vi "op_ClearNoise.vi"(0 "EQ folder path Refnum":refnum<vi>, 1 "HV enable button":bool caption="High Voltage enable", 2 "HV parameters Refnum":refnum<vi>, 3 "HV level Refnum":refnum<vi>, 4 "HV string Refnum":refnum<vi>, 5 "Stop ACQ button Refnum":refnum<vi>, 6 "ACQ Parameters (cluster)":T3={"Acquisition Mode"=0, "Pulse width"=0, "DTP period"=1, "Number of events"=4000} caption="Acquisition Parameters" {"Number of events" min=1; "DTP period" min=1; "Pulse width" items=["25 ns", "50 ns", "75 ns", "100 ns"]; "Acquisition Mode" items=["Normal", "Pedestal", "Test Pulse", "Test Pulse trigger & synchronous"]}, 7 "Events to acquire Refnum":refnum<vi>, 8 "error tick Refnum":refnum<vi>, 9 "ACQ events fets Refnum":refnum<vi>, 10 "Operation text Refnum":refnum<vi>, 11 "ACQ events fets A Refnum":refnum<vi>, 12 "Busy Refnum":refnum<vi>, 13 "ACQ events fets B Refnum":refnum<vi>, 14 "Addresses Cluster":T2={"ENA1"=FALSE, "IP address 1"="172.16.14.22", "ENA2"=FALSE, "IP address 2"="172.16.14.23"}, 15 "etapa# terminals refnums":T4, 17 "GbReg params":u8[](array[numeric])=[32, 22], 19 "LayerChipIDs":u16[](array[numeric])=[65535, 65535] format="%04x", 27 "ClearNoise vars":T1={"Waiting time X"=100, "ClearNoise ACQits"=2, "Threshold Z"=1000, "HVit Refnum"=refnum, "ACQit Refnum"=refnum} {"ClearNoise ACQits" min=1 step=1}) -> (23 "Folder path: acquisition reports":path=path "C:/VIPauto/Files/LayerID/Acquisition/yyyymmdd_hh-mm-ss_Leak#_HV#")   [LabVIEW 2015, in "VIPM2.lvlib"]
uses:
  VIPM2.lvlib
panel:
  out "Chip ID list 1":u32[](array[numeric]) format="%.0x"
  out "Layer ID list 1 (ordered)":u32[](array[numeric]) format="%.0x"
  out "All ID list 1":u32[](array[numeric]) format="%.0x"
  out "Chip ID list 2":u32[](array[numeric]) format="%.0x"
  out "Layer ID list 2 (ordered)":u32[](array[numeric]) format="%.0x"
  out "All ID list 2":u32[](array[numeric]) format="%.0x"
  # "Operation: ClearNoise, with HV (refnums)"
  # "Analog Vref low"
  # "Gb THLD"
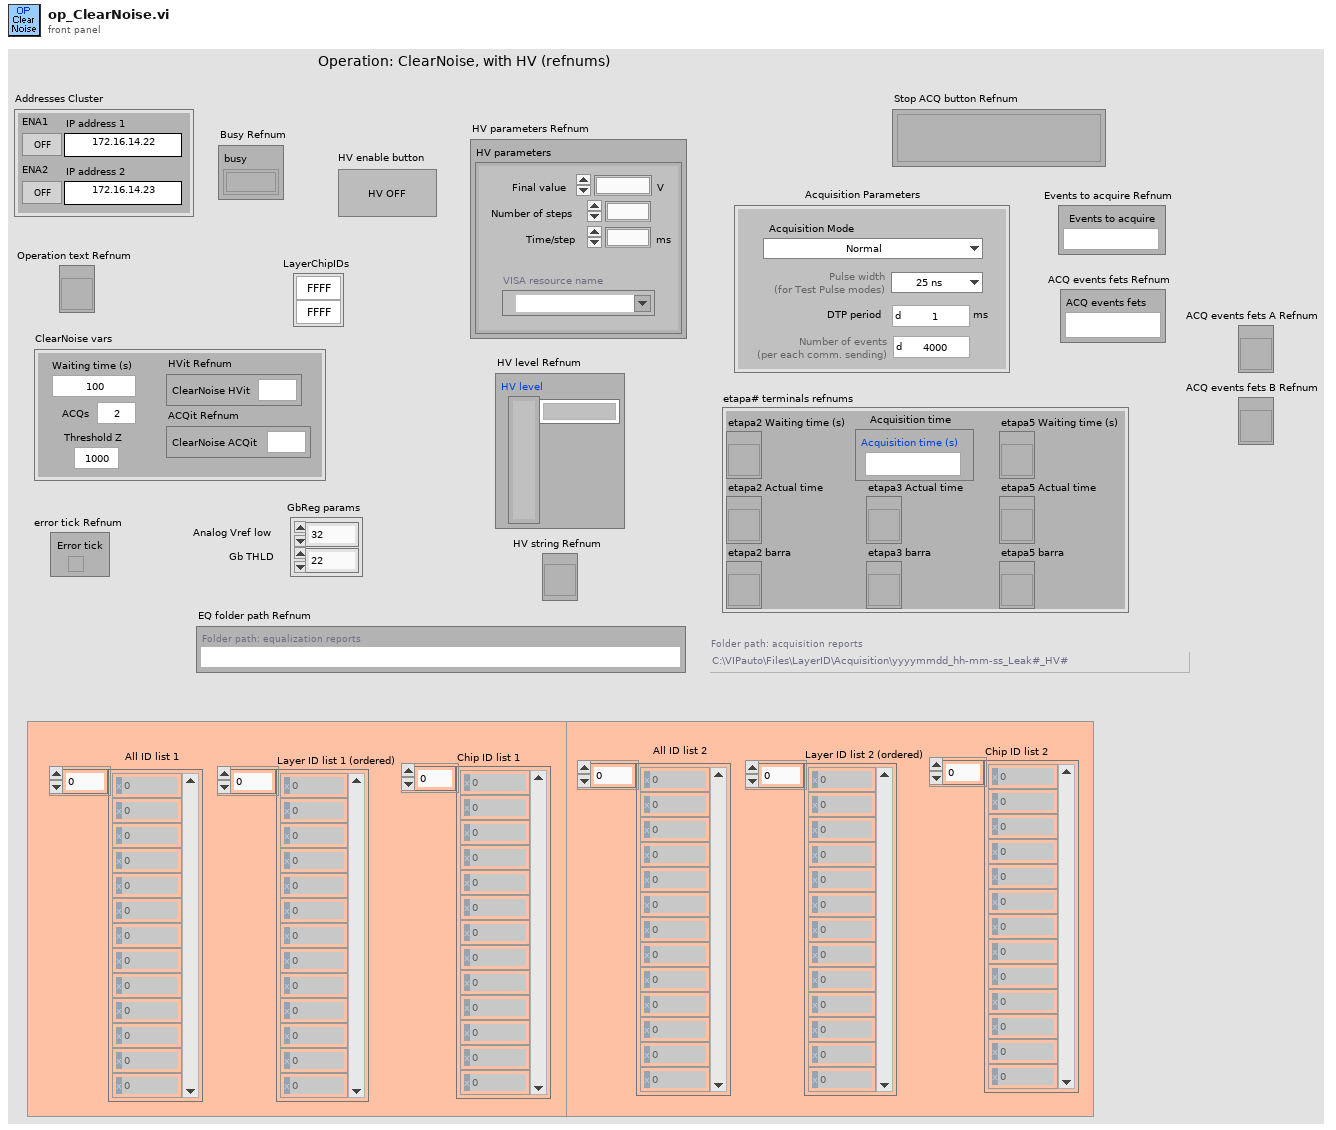
[diagram p1: front panel]
types:
  T1 = cluster{"Waiting time X":u32, "ClearNoise ACQits":i32, "Threshold Z":u32, "HVit Refnum":refnum<vi>, "ACQit Refnum":refnum<vi>}
  T2 = cluster{"ENA1":bool, "IP address 1":string, "ENA2":bool, "IP address 2":string}
  T3 = cluster{"Acquisition Mode":u32, "Pulse width":u32, "DTP period":u32, "Number of events":u32}
  T4 = cluster{"etapa2 Waiting time (s)":refnum<vi>, "etapa2 Actual time":refnum<vi>, "etapa2 barra":refnum<vi>, "etapa3 Actual time":refnum<vi>, "etapa3 barra":refnum<vi>, "etapa5 Waiting time (s)":refnum<vi>, "etapa5 Actual time":refnum<vi>, "etapa5 barra":refnum<vi>, "Acquisition time":refnum<vi>}
  T5 = enum8{"Enabled", "Disabled", "Disabled and Grayed Out"}
  T6 = cluster{"Final value":i16, "Number of steps":u8, "Time/step":u16, "Output Off Behavior":u16, "VISA resource name":refnum<visa-resource-name>}
  T7 = cluster{"ChipID":u16, "Hot pixels to kill":u8[]}[]
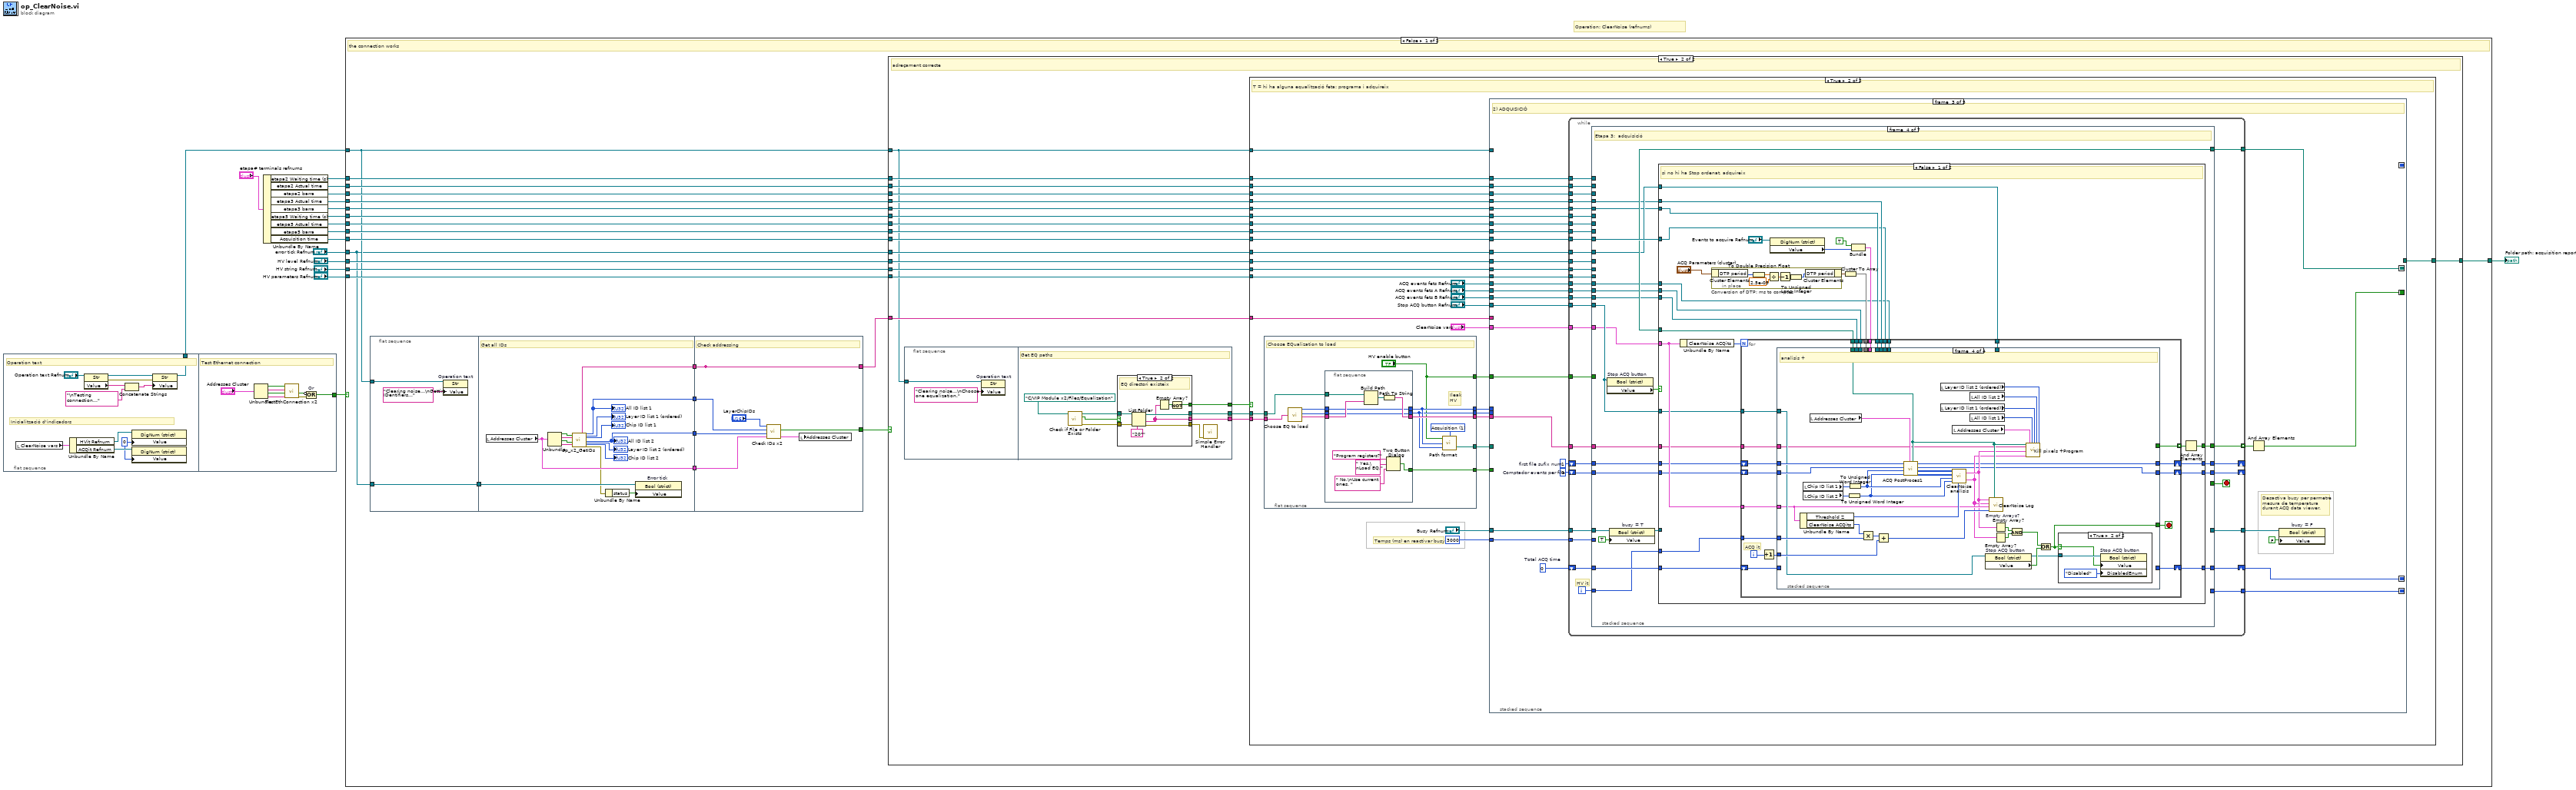
[diagram p0: block diagram]
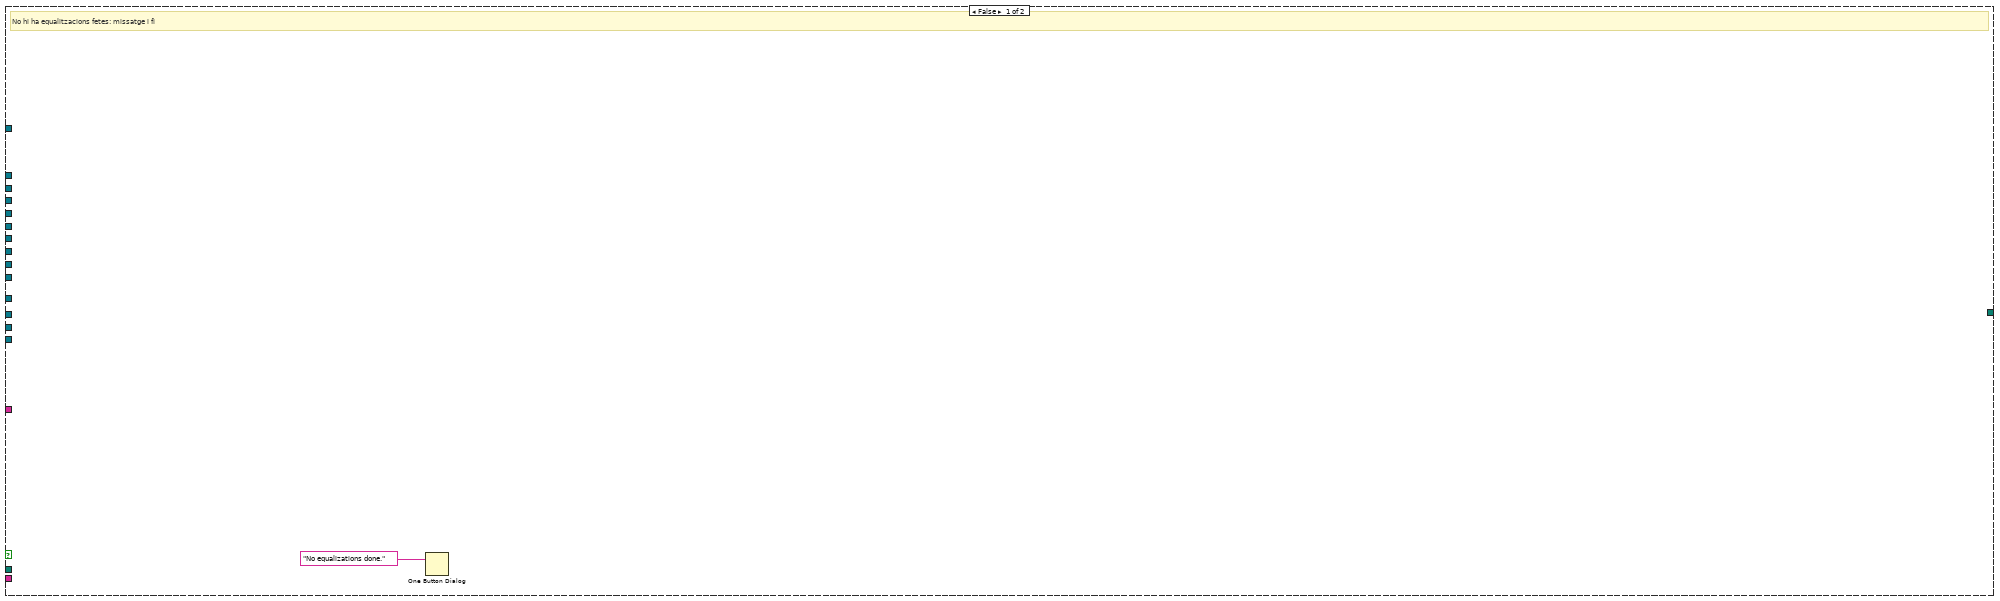
[diagram p4: hidden frame]
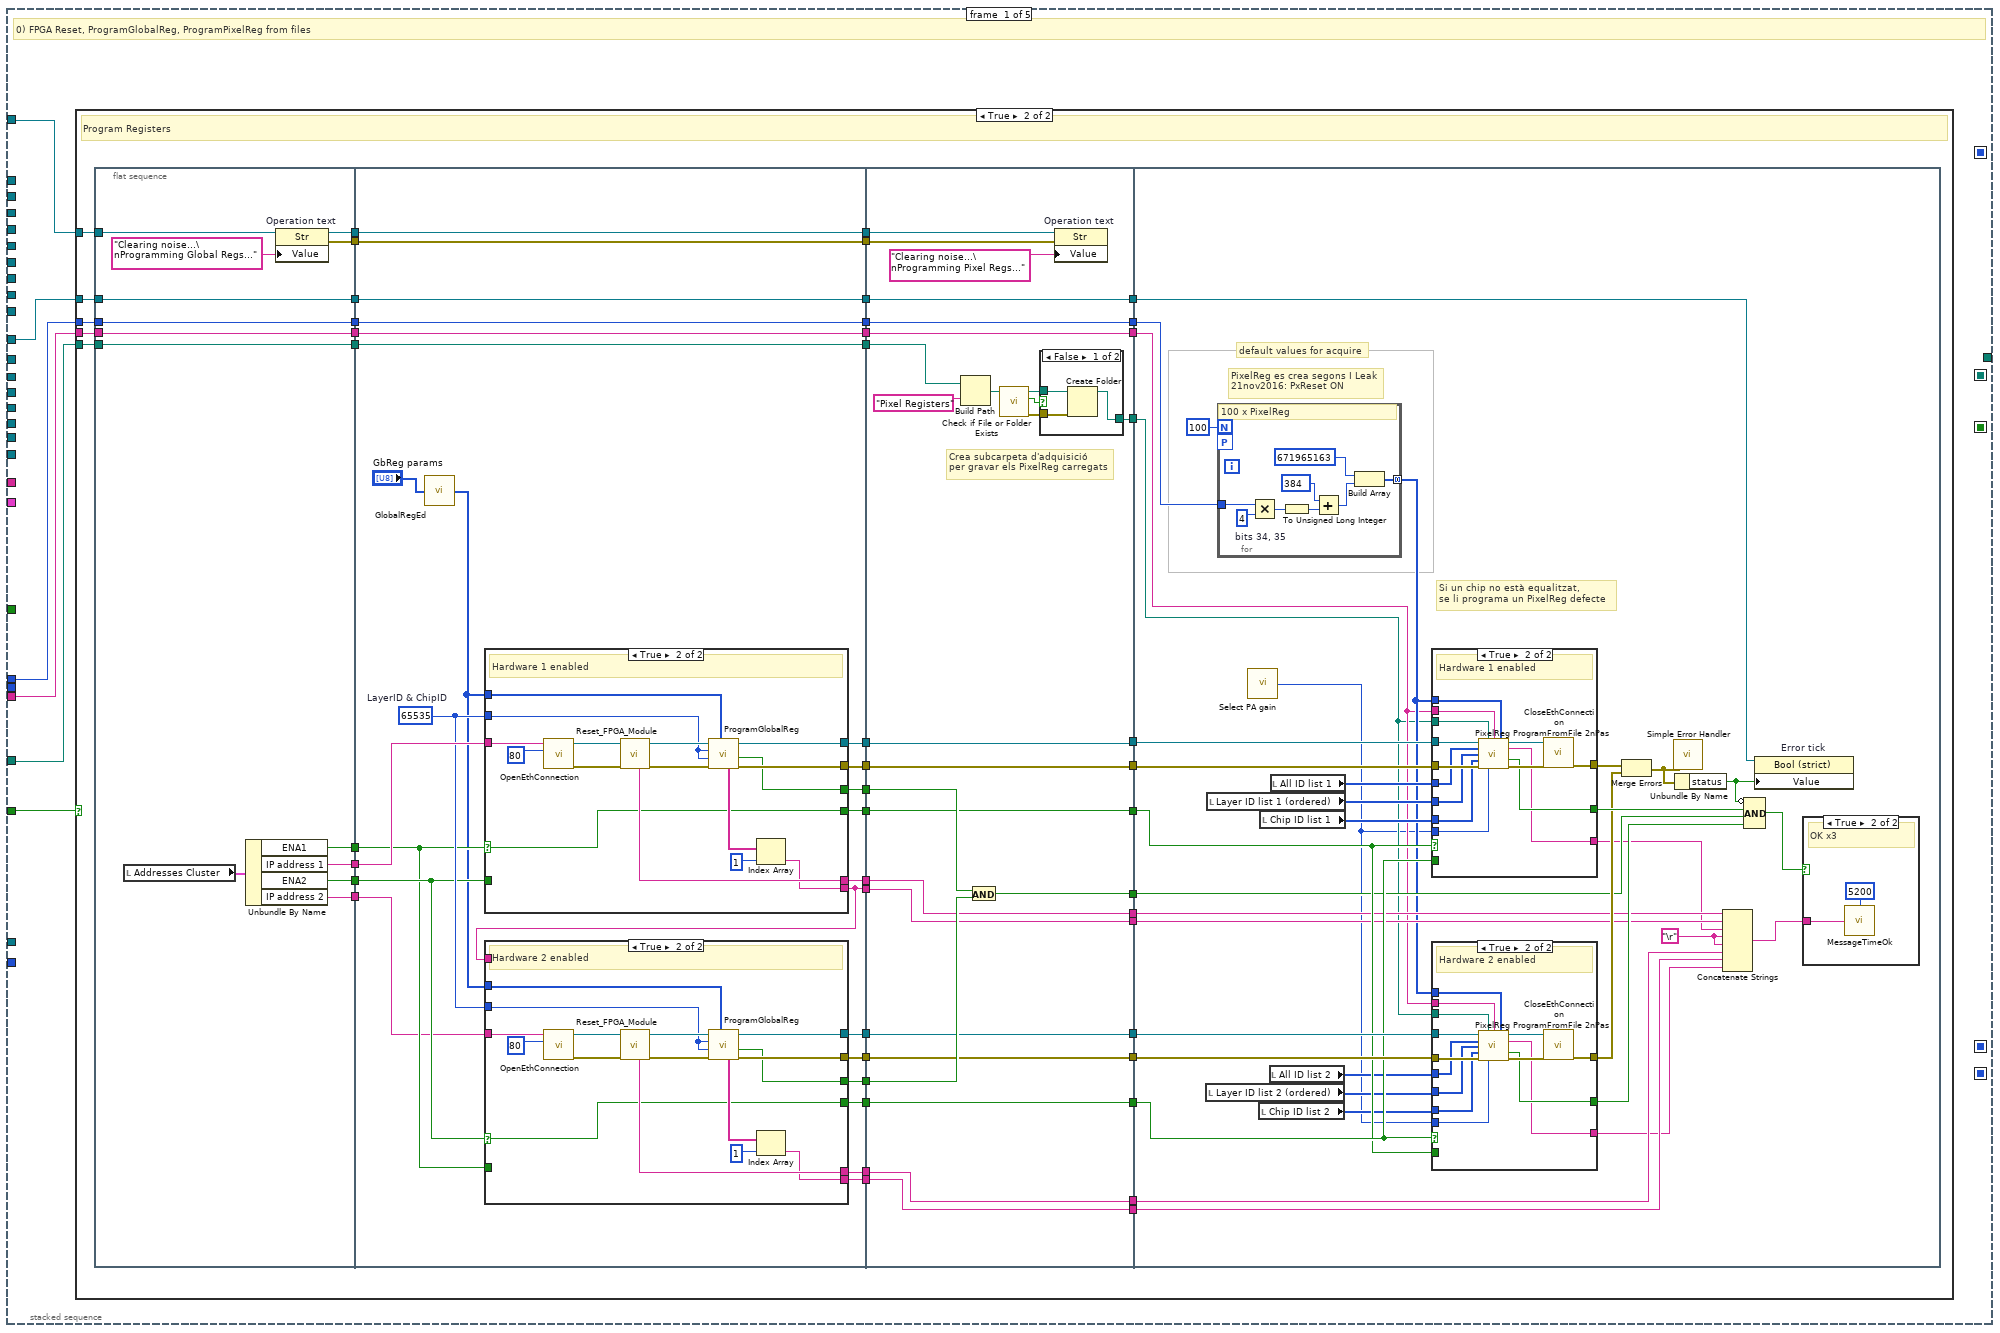
[diagram p5: hidden frame]
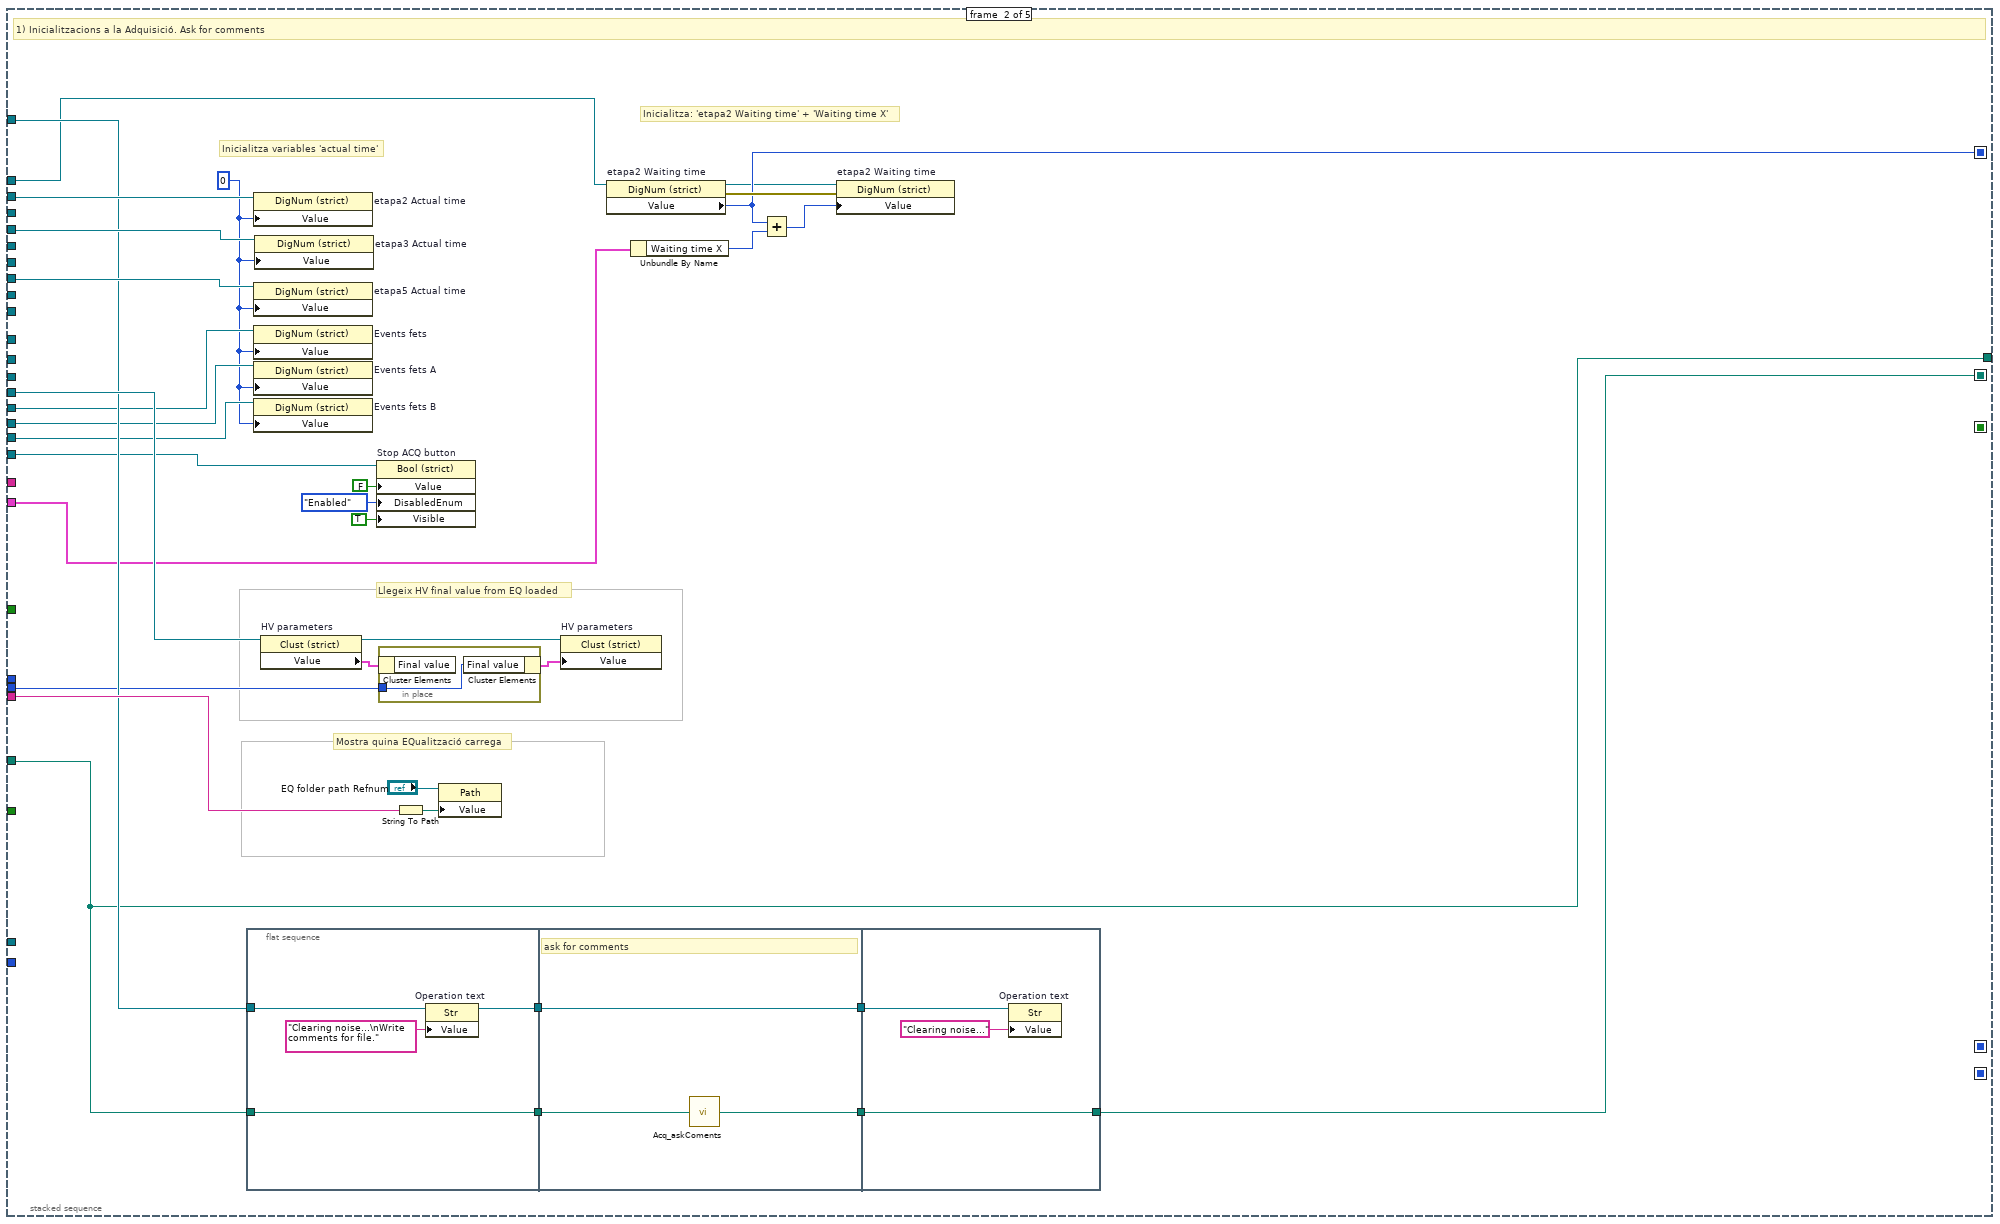
[diagram p13: hidden frame]
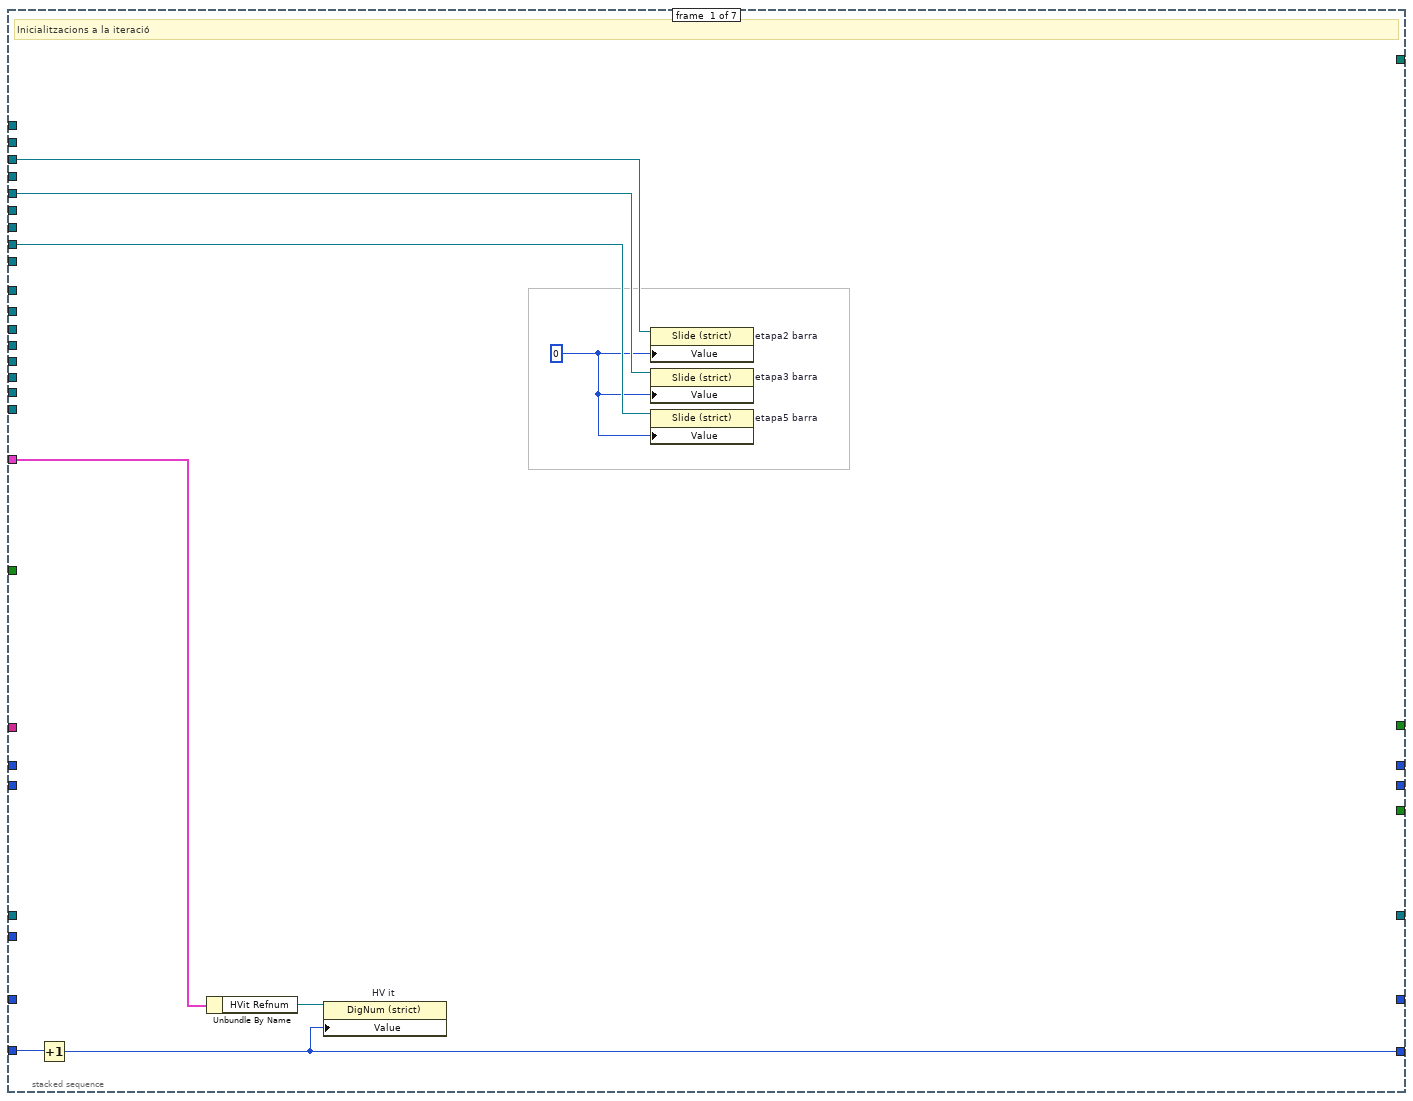
[diagram p14: hidden frame]
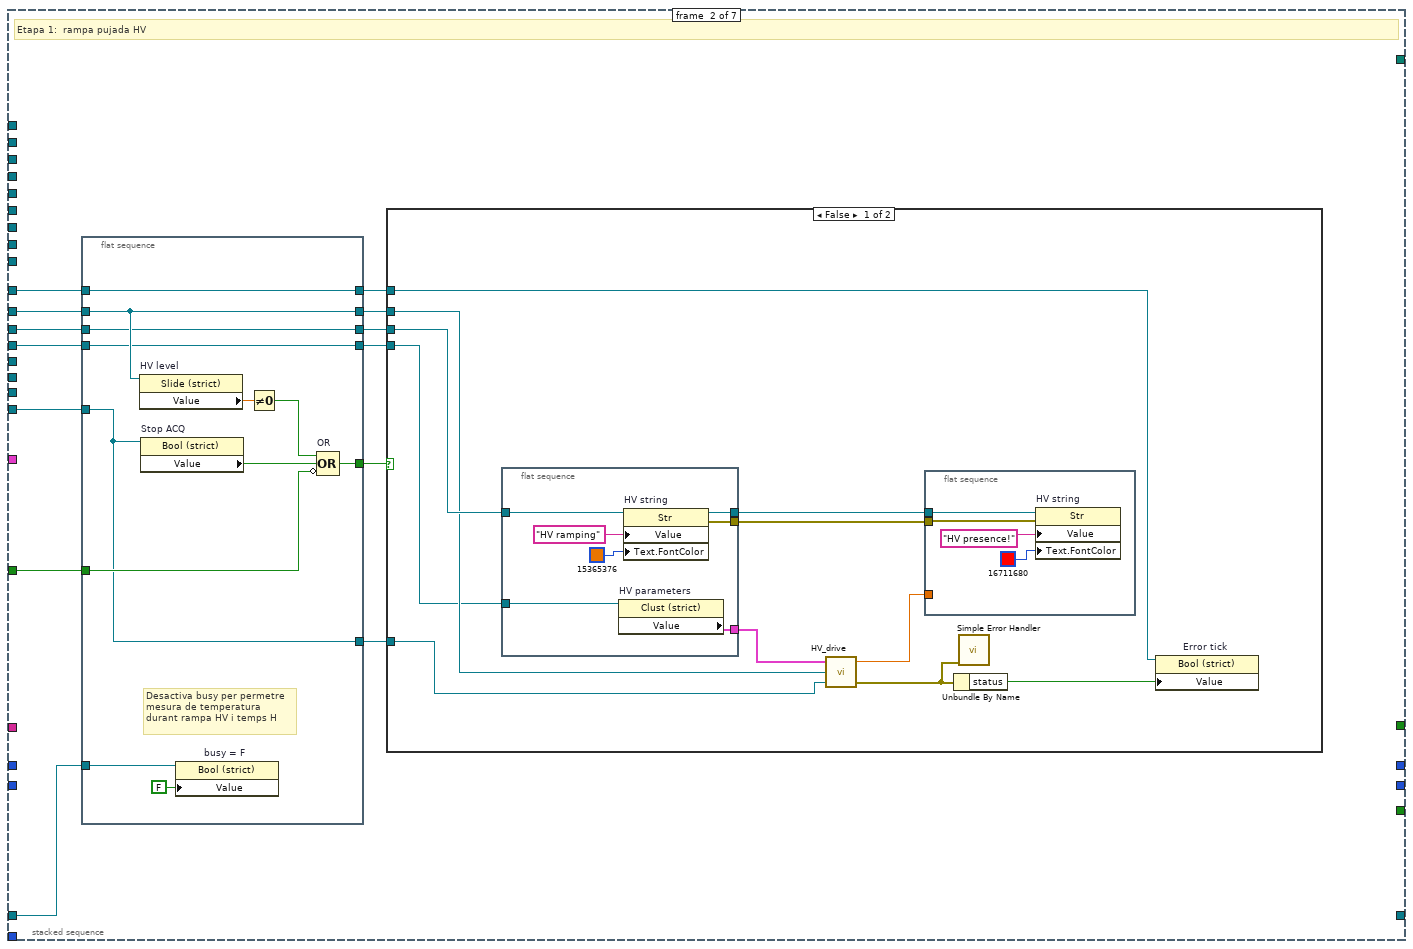
[diagram p15: hidden frame]
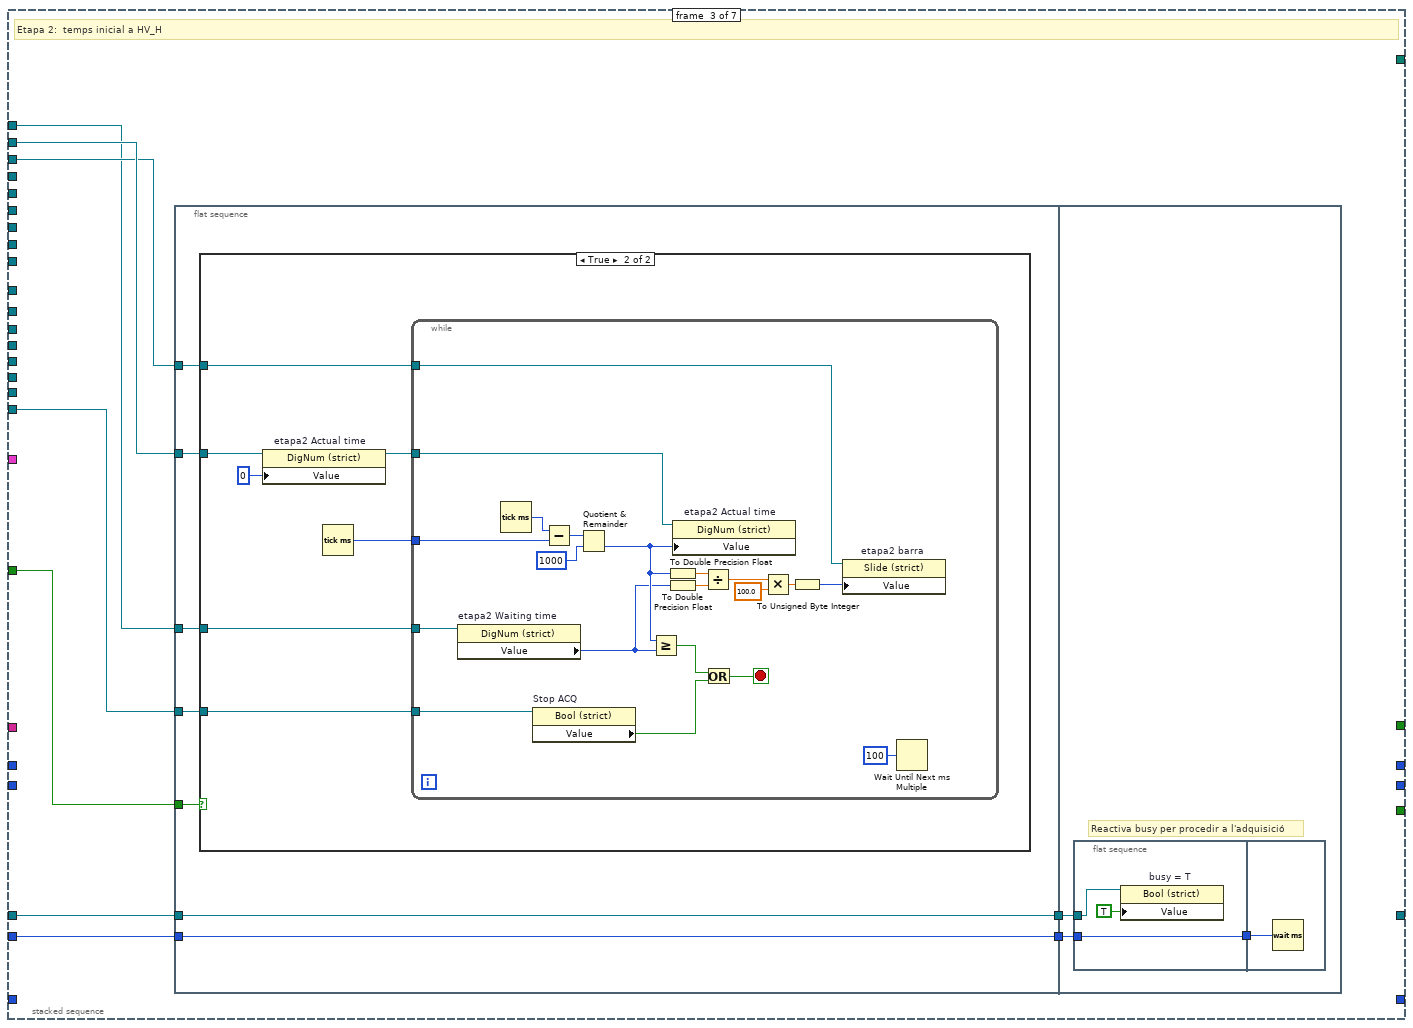
[diagram p17: hidden frame]
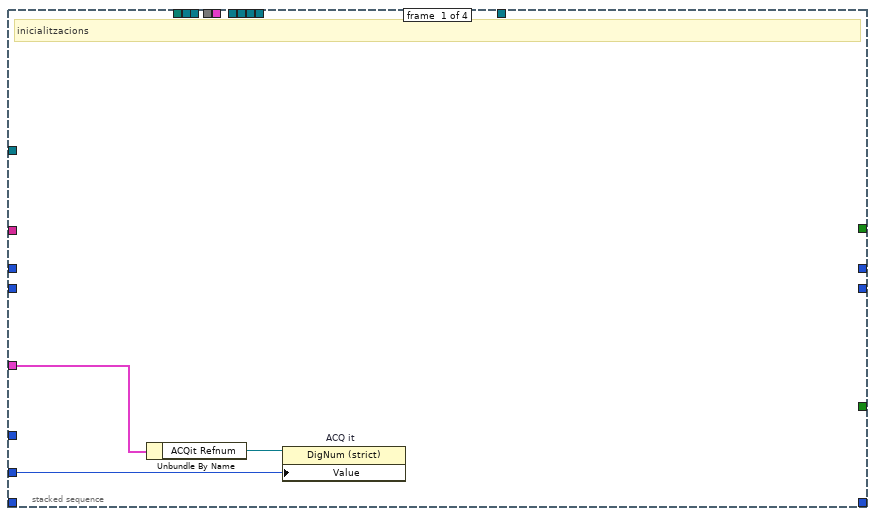
[diagram p19: hidden frame]
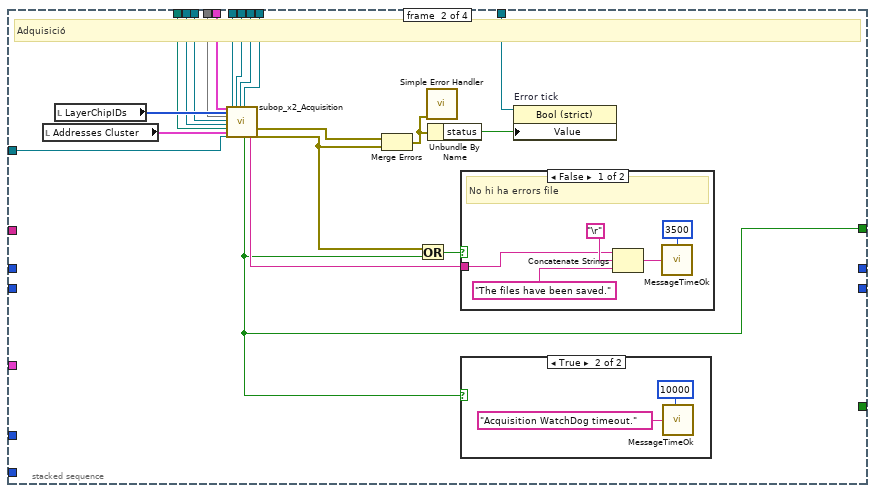
[diagram p20: hidden frame]
diagram:
  # "Operation: ClearNoise (refnums)"
  n1 = flat-sequence {
    tunnel: [w22] -> w7
    tunnel: [w34] -> w17
    frame #0 {
      w18 = 0 ("Value")
      # "Inicialització d'indicadors"
      # "Operation text"
      n2 = local read "ClearNoise vars"() -> (w21:T1)
      n3 = Unbundle By Name(w21) -> ("HVit Refnum"=w19:refnum<vi>, "ACQit Refnum"=w20:refnum<vi>)
      n4 = property class="Str"(reference="Operation text Refnum") -> (reference out=w25:refnum<vi>, error out=w24:errorcluster, "Value"=w27:string)  [unwired: 1 in]
      n5 = Concatenate Strings "Concatenate Strings"(w27, "\nTesting connection..." ("string")) -> (w23:string)
      n6 = property class="DigNum (strict)"(reference=w19, "Value"=w18) -> ()  [unwired: 1 in, 2 out]
      n7 = property class="DigNum (strict)"(reference=w20, "Value"=w18) -> ()  [unwired: 1 in, 2 out]
      n8 = property class="Str"(reference=w25, error in=w24, "Value"=w23) -> (reference out=w22:refnum<vi>)  [unwired: 1 out]
    }
    frame #1 {
      # "Test Ethernet connection"
      n9 = Unbundle("Addresses Cluster") -> ("ENA1"=w32:bool, "IP address 1"=w31:string, "ENA2"=w30:bool, "IP address 2"=w29:string)
      n10 = call "TestEthConnection x2.vi"("IP address 2"=w29, "ENA2"=w30, "IP address 1"=w31, "ENA1"=w32) -> ("error out"=w35:errorcluster, "Answers OK?"=w36:bool)  [unwired: 6 in]
      n11 = Compound Arithmetic op=OR "Or"(invert w36, w35) -> (w34:bool)
    }
  }
  n12 = Unbundle By Name("etapa# terminals refnums") -> ("etapa2 Waiting time (s)"=w15:refnum<vi>, "etapa2 Actual time"=w14:refnum<vi>, "etapa2 barra"=w13:refnum<vi>, "etapa3 Actual time"=w12:refnum<vi>, "etapa3 barra"=w11:refnum<vi>, "etapa5 Waiting time (s)"=w10:refnum<vi>, "etapa5 Actual time"=w9:refnum<vi>, "etapa5 barra"=w8:refnum<vi>, "Acquisition time"=w2:refnum<vi>)
  n13 = case shown="False" w17 {
    selector: w17 -> [_ w954]
    tunnel: w15 -> [w58 _]
    tunnel: w14 -> [w57 _]
    tunnel: w13 -> [w56 _]
    tunnel: w12 -> [w55 _]
    tunnel: w11 -> [w54 _]
    tunnel: w10 -> [w53 _]
    tunnel: w9 -> [w52 _]
    tunnel: w8 -> [w51 _]
    tunnel: w7 -> [w40 _]
    tunnel: "HV level Refnum" -> [w50 _]
    tunnel: "HV string Refnum" -> [w49 _]
    tunnel: "error tick Refnum" -> [w39 w953]
    tunnel: [w48 _] -> w1
    tunnel: "HV parameters Refnum" -> [w47 _]
    tunnel: w2 -> [w46 _]
    frame False {
      # "the connection works"
      n14 = flat-sequence {
        tunnel: w40 -> [w930]
        tunnel: w39 -> [w928]
        tunnel: [w928] -> w45
        tunnel: w45 -> [w936]
        tunnel: [w935] -> w44
        tunnel: [w934] -> w43
        tunnel: [w933] -> w42
        tunnel: [w932] -> w41
        tunnel: [w946] -> _
        tunnel: w44 -> [w946]
        tunnel: w43 -> [w950]
        tunnel: w42 -> [w951]
        tunnel: w41 -> [w952]
        tunnel: [w948] -> w38
        tunnel: [w946] -> w37
        frame #0 {
          n15 = property on="Operation text" class="Str"(reference=w930, "Value"="Clearing noise...\nGetting IDentifiers...") -> ()  [unwired: 1 in, 2 out]
        }
        frame #1 {
          # "Get all IDs"
          n16 = local read "Addresses Cluster"() -> (w932:T2)
          n17 = Unbundle(w932) -> ("ENA1"=w938:bool, "IP address 1"=w939:string, "ENA2"=w941:bool, "IP address 2"=w940:string)
          n18 = call "op_x2_GetIDs.vi"("ENA1"=w938, "IP address 1"=w939, "ENA2"=w941, "IP address 2"=w940) -> ("summary IDs"=w935:string, "All ID list 1"=w934:u32[], "Layer ID list 1 (ordered)"=→"Layer ID list 1 (ordered)":u32[], "Chip ID list 1"=→"Chip ID list 1":u32[], "All ID list 2"=w933:u32[], "Layer ID list 2 (ordered)"=→"Layer ID list 2 (ordered)":u32[], "Chip ID list 2"=→"Chip ID list 2":u32[], "error out"=w931:errorcluster)  [unwired: 16 in]
          "All ID list 1" <- w934
          "All ID list 2" <- w933
          n19 = Unbundle By Name(w931) -> ("status"=w937:bool)
          n20 = property on="Error tick" class="Bool (strict)"(reference=w936, "Value"=w937) -> ()  [unwired: 1 in, 2 out]
        }
        frame #2 {
          # "Check addressing"
          n21 = call "Check IDs x2.vi"("Addresses Cluster in"=w952, "All ID list 2"=w951, "All ID list 1"=w950, "LayerChipIDs"="LayerChipIDs") -> ("Addresses Cluster out"=w949:T2, "OK?"=w948:bool)  [unwired: 6 in]
          n22 = local write "Addresses Cluster"(w949) -> ()
        }
      }
      n23 = case shown="True" w38 {
        tunnel: w58 -> [_ w77]
        tunnel: w57 -> [_ w76]
        tunnel: w56 -> [_ w75]
        tunnel: w55 -> [_ w74]
        tunnel: w54 -> [_ w73]
        tunnel: w53 -> [_ w72]
        tunnel: w52 -> [_ w71]
        tunnel: w51 -> [_ w70]
        tunnel: w50 -> [_ w69]
        tunnel: w49 -> [_ w68]
        tunnel: [_ w67] -> w48
        tunnel: w47 -> [_ w66]
        tunnel: w46 -> [_ w65]
        tunnel: w40 -> [_ w59]
        tunnel: w39 -> [_ w64]
        tunnel: w37 -> [_ w60]
        frame False {
          # "adreçament incorrecte"
        }
        frame True {
          # "adreçament correcte"
          n24 = flat-sequence {
            tunnel: w59 -> [w78]
            tunnel: [w87] -> w61
            tunnel: [w86] -> w62
            tunnel: [w85] -> w63
            frame #0 {
              n25 = property on="Operation text" class="Str"(reference=w78, "Value"="Clearing noise...\nChoose one equalization.") -> ()  [unwired: 1 in, 2 out]
            }
            frame #1 {
              # "Get EQ paths"
              n26 = call <vilib>:"Check if File or Folder Exists.vi"("path"=path "C:/VIP Module x2/Files/Equalization") -> ("error out"=w81:errorcluster, "file or folder exists?"=w82:bool, "dup path"=w83:path)  [unwired: 8 in]
              n27 = case shown="True" w82 {
                selector: w82 -> [w90 _]
                tunnel: w83 -> [w89 w96]
                tunnel: w81 -> [w88 w95]
                tunnel: [w90 w92] -> w87
                tunnel: [w89 w93] -> w86
                tunnel: [w88 w94] -> w80
                tunnel: [_ w91] -> w85
                frame False {
                  # "no EQs"
                }
                frame True {
                  # "EQ directori existeix"
                  n28 = List Folder(path=w96, pattern="20*", error in=w95) -> (path out=w93:path, folder names=w91:string[], error out=w94:errorcluster)  [unwired: 1 in, 1 out]
                  n29 = Empty Array?(array=w91) -> (empty?=w97:bool)
                  n30 = Not(x=w97) -> (.not. x?=w92:bool)
                }
              }
              n31 = call <vilib>:"Simple Error Handler.vi"("error in (no error)"=w80) -> ()  [unwired: 4 in, 5 out]
            }
          }
          n32 = case shown="True" w61 {
            tunnel: w77 -> [_ w130]
            tunnel: w76 -> [_ w129]
            tunnel: w75 -> [_ w128]
            tunnel: w74 -> [_ w127]
            tunnel: w73 -> [_ w126]
            tunnel: w72 -> [_ w125]
            tunnel: w71 -> [_ w124]
            tunnel: w70 -> [_ w123]
            tunnel: w69 -> [_ w122]
            tunnel: w68 -> [_ w121]
            tunnel: [_ w120] -> w67
            tunnel: w59 -> [_ w119]
            tunnel: w64 -> [_ w118]
            tunnel: w62 -> [_ w117]
            tunnel: w63 -> [_ w116]
            tunnel: w66 -> [_ w112]
            tunnel: w65 -> [_ w109]
            tunnel: w60 -> [_ w107]
            frame False {
              # "No hi ha equalitzacions fetes: missatge i fi"
              n33 = One Button Dialog(message="No equalizations done.") -> ()  [unwired: 1 in, 1 out]
            }
            frame True {
              # "Temps (ms) en reactivar busy"
              # "T = hi ha alguna equalització feta: programa i adquireix"
              n34 = flat-sequence {
                tunnel: w117 -> [w139]
                tunnel: w116 -> [w140]
                tunnel: [w137] -> w115
                tunnel: [w132] -> w114
                tunnel: [w135] -> w113
                tunnel: [w141] -> w111
                tunnel: [w136] -> w106
                tunnel: ["HV enable button"] -> w103
                frame #0 {
                  w142 = u8 1 items=["Equalization", "Acquisition"] ("Operation type")
                  # "Ileak\nHV"
                  # "Choose EQualization to load"
                  n35 = call "Choose EQ to load.vi"("EQ folders"=w140) -> ("I Leakage"=w134:u8, "HV last value"=w133:i16, "loaded EQ folder"=w138:string)  [unwired: 5 in]
                  n36 = flat-sequence {
                    tunnel: w139 -> [w152]
                    tunnel: w138 -> [w151]
                    tunnel: [w149] -> w137
                    tunnel: [w148] -> w136
                    tunnel: [w144] -> w135
                    tunnel: w134 -> [w144]
                    tunnel: w133 -> [w143]
                    tunnel: [w143] -> w132
                    frame #0 {
                      n37 = Build Path(base path=w152, name or relative path=w151) -> (appended path=w150:path)
                      n38 = Path To String(path=w150) -> (string=w149:string)
                      n39 = Two Button Dialog(message="Program registers?", 1:" No.\nUse current ones. " ("F button name (\"Cancel\")"), 2:" Yes.\nLoad EQ." ("T button name (\"OK\")")) -> (T button?=w148:bool)
                    }
                  }
                  n40 = call "Path format.vi"("Operation type"=w142, "HV level"=w132, "I leakage"=w135, "HV enable button"="HV enable button") -> ("folder path"=w141:path)  [unwired: 1 in]
                }
              }
              n41 = stacked-sequence {
                seq-local: [_ _ w433 _ _] -> [_ _ _ _ w880]
                seq-local: [_ w405 _ _ _] -> [_ _ w449 _ w879]
                seq-local: [_ _ w441 _ _] -> [_ _ _ _ w859]
                seq-local: [_ _ w439 _ _] -> [_ _ _ _ w858]
                seq-local: [_ w391 _ _ _] -> [_ _ _ w853 _]
                tunnel: w119 -> [w158 w410 _ _ w877]
                tunnel: w130 -> [_ w394 w463 w854 w860]
                tunnel: w129 -> [_ w420 w462 _ _]
                tunnel: w128 -> [_ _ w461 _ _]
                tunnel: w127 -> [_ w419 w460 _ _]
                tunnel: w126 -> [_ _ w459 _ _]
                tunnel: w125 -> [_ _ w458 _ w861]
                tunnel: w124 -> [_ w418 w457 _ _]
                tunnel: w123 -> [_ _ w456 _ _]
                tunnel: w118 -> [w157 _ w453 _ _]
                tunnel: w122 -> [_ _ w455 _ _]
                tunnel: w121 -> [_ _ w454 _ _]
                tunnel: [_ w403 _ _ _] -> w120
                tunnel: w115 -> [w156 w411 w432 _ w865]
                tunnel: w114 -> [_ w409 _ _ _]
                tunnel: w113 -> [w155 _ _ _ _]
                tunnel: w112 -> [_ w417 w452 _ w863]
                tunnel: w111 -> [w154 w403 _ _ w866]
                tunnel: "Stop ACQ button Refnum" -> [_ w402 w451 w857 _]
                tunnel: w109 -> [_ _ w450 _ w862]
                tunnel: "ACQ events fets Refnum" -> [_ w398 w448 _ w864]
                tunnel: w107 -> [_ _ _ _ w878]
                tunnel: w106 -> [w153 _ _ _ w867]
                tunnel: "Busy Refnum" -> [_ _ w447 _ _]
                tunnel: u32 3000 -> [_ _ w446 _ _]
                tunnel: w103 -> [_ _ w442 _ _]
                tunnel: "ACQ events fets A Refnum" -> [_ w397 w438 _ _]
                tunnel: "ACQ events fets B Refnum" -> [_ w396 w437 _ _]
                tunnel: "ClearNoise vars" -> [_ w393 w435 _ _]
                frame #0 {
                  # "0) FPGA Reset, ProgramGlobalReg, ProgramPixelReg from files"
                  n42 = case shown="True" w153 {
                    tunnel: w158 -> [_ w189]
                    tunnel: w157 -> [_ w188]
                    tunnel: w156 -> [_ w187]
                    tunnel: w155 -> [_ w186]
                    tunnel: w154 -> [_ w185]
                    frame False {
                      # "Use current registers values"
                    }
                    frame True {
                      # "Program Registers"
                      n43 = flat-sequence {
                        tunnel: w189 -> [w218]
                        tunnel: [w217] -> w206
                        tunnel: [w216] -> w205
                        tunnel: [w215] -> w204
                        tunnel: w188 -> [w215]
                        tunnel: [w214] -> w203
                        tunnel: w187 -> [w214]
                        tunnel: [w213] -> w202
                        tunnel: w186 -> [w213]
                        tunnel: [w212] -> w201
                        tunnel: w185 -> [w212]
                        tunnel: [w210] -> w184
                        tunnel: [w209] -> w183
                        tunnel: [w208] -> w182
                        tunnel: [w207] -> w181
                        tunnel: w206 -> [w244]
                        tunnel: w205 -> [w243]
                        tunnel: [w244] -> w200
                        tunnel: [w243] -> w199
                        tunnel: [w242] -> w198
                        tunnel: w204 -> [w242]
                        tunnel: w203 -> [w241]
                        tunnel: [w241] -> w197
                        tunnel: w202 -> [w240]
                        tunnel: [w240] -> w196
                        tunnel: w201 -> [w239]
                        tunnel: [w239] -> w195
                        tunnel: w184 -> [w235]
                        tunnel: w183 -> [w236]
                        tunnel: w182 -> [w238]
                        tunnel: w181 -> [w234]
                        tunnel: [w233] -> w180
                        tunnel: [w232] -> w179
                        tunnel: [w231] -> w178
                        tunnel: [w230] -> w177
                        tunnel: [w229] -> w176
                        tunnel: [w222] -> w175
                        tunnel: [w228] -> w174
                        tunnel: [w227] -> w173
                        tunnel: [w226] -> w172
                        tunnel: [w225] -> w171
                        tunnel: [w224] -> w170
                        tunnel: [w223] -> w169
                        tunnel: w200 -> [w305]
                        tunnel: w199 -> [w304]
                        tunnel: [w291] -> w194
                        tunnel: [w290] -> w193
                        tunnel: [w303] -> w192
                        tunnel: w198 -> [w303]
                        tunnel: [w302] -> w191
                        tunnel: w197 -> [w302]
                        tunnel: [w301] -> w190
                        tunnel: w196 -> [w301]
                        tunnel: w195 -> [w293]
                        tunnel: w180 -> [w291]
                        tunnel: w179 -> [w290]
                        tunnel: w178 -> [w300]
                        tunnel: w177 -> [w289]
                        tunnel: w176 -> [w284]
                        tunnel: w175 -> [w283]
                        tunnel: w174 -> [w288]
                        tunnel: w173 -> [w287]
                        tunnel: w172 -> [w299]
                        tunnel: w171 -> [w286]
                        tunnel: w170 -> [w282]
                        tunnel: w169 -> [w281]
                        tunnel: [w292] -> w168
                        tunnel: [w289] -> w167
                        tunnel: [w288] -> w166
                        tunnel: [w287] -> w165
                        tunnel: [w286] -> w164
                        tunnel: [w285] -> w163
                        tunnel: [w284] -> w162
                        tunnel: [w283] -> w161
                        tunnel: [w282] -> w160
                        tunnel: [w281] -> w159
                        tunnel: w194 -> [w340]
                        tunnel: w193 -> [w339]
                        tunnel: w192 -> [w342]
                        tunnel: w191 -> [w318]
                        tunnel: w190 -> [w337]
                        tunnel: w168 -> [w317]
                        tunnel: w167 -> [w330]
                        tunnel: w166 -> [w333]
                        tunnel: w165 -> [w332]
                        tunnel: w164 -> [w331]
                        tunnel: w163 -> [w323]
                        tunnel: w162 -> [w321]
                        tunnel: w161 -> [w320]
                        tunnel: w160 -> [w314]
                        tunnel: w159 -> [w313]
                        frame #0 {
                          n44 = local read "Addresses Cluster"() -> (w211:T2)
                          n45 = Unbundle By Name(w211) -> ("ENA1"=w210:bool, "IP address 1"=w208:string, "ENA2"=w209:bool, "IP address 2"=w207:string)
                          n46 = property on="Operation text" class="Str"(reference=w218, "Value"="Clearing noise...\nProgramming Global Regs...") -> (reference out=w217:refnum<vi>, error out=w216:errorcluster)  [unwired: 1 in]
                        }
                        frame #1 {
                          w237 = u32 65535  # LayerID & ChipID
                          n47 = call "GlobalRegEd.vi"("params"="GbReg params") -> ("Global Reg out"=w221:u32[])  [unwired: 4 in]
                          n48 = case shown="True" w235 {
                            selector: w235 -> [w264 w265]
                            tunnel: w237 -> [_ w267]
                            tunnel: [_ w273] -> w233
                            tunnel: [_ w272] -> w232
                            tunnel: [_ w271] -> w229
                            tunnel: [_ w270] -> w222
                            tunnel: [w263 w269] -> w231
                            tunnel: w221 -> [_ w268]
                            tunnel: w238 -> [_ w266]
                            tunnel: [w264 w265] -> w230
                            tunnel: w236 -> [w263 _]
                            frame False {
                              # "Hardware 1 not enabled"
                            }
                            frame True {
                              # "Hardware 1 enabled"
                              n49 = call "OpenEthConnection.vi"("Port"=u16 80, "IP address"=w266) -> ("error out"=w279:errorcluster, "connection ID out"=w280:refnum<k5>)  [unwired: 7 in, 1 out]
                              n50 = call "Reset_FPGA_Module.vi"("error in (no error)"=w279, "connection ID"=w280) -> ("error out"=w276:errorcluster, "connection ID out"=w277:refnum<k5>, "Answer to Reset"=w271:string)  [unwired: 7 in]
                              n51 = call "ProgramGlobalReg.vi"("Global Reg"=w268, "error in (no error)"=w276, "ChipID"=w267, "LayerID"=w267, "connection ID"=w277) -> ("error out"=w272:errorcluster, "OK?"=w269:bool, "connection ID out"=w273:refnum<k5>, "Program done"=w275:string[])  [unwired: 2 in, 1 out]
                              n52 = Index Array "Index Array"(array=w275, index=1) -> (element=w270:string)
                            }
                          }
                          n53 = case shown="True" w236 {
                            selector: w236 -> [w246 w247]
                            tunnel: w237 -> [_ w249]
                            tunnel: [_ w255] -> w228
                            tunnel: [_ w254] -> w227
                            tunnel: [_ w253] -> w224
                            tunnel: [_ w252] -> w223
                            tunnel: [w245 w251] -> w226
                            tunnel: w221 -> [_ w250]
                            tunnel: w234 -> [_ w248]
                            tunnel: [w246 w247] -> w225
                            tunnel: w235 -> [w245 _]
                            tunnel: w222 -> [_ _]
                            frame False {
                              # "Hardware 2 not enabled"
                            }
                            frame True {
                              # "Hardware 2 enabled"
                              n54 = call "OpenEthConnection.vi"("Port"=u16 80, "IP address"=w248) -> ("error out"=w261:errorcluster, "connection ID out"=w262:refnum<k5>)  [unwired: 7 in, 1 out]
                              n55 = call "Reset_FPGA_Module.vi"("error in (no error)"=w261, "connection ID"=w262) -> ("error out"=w258:errorcluster, "connection ID out"=w259:refnum<k5>, "Answer to Reset"=w253:string)  [unwired: 7 in]
                              n56 = call "ProgramGlobalReg.vi"("Global Reg"=w250, "error in (no error)"=w258, "ChipID"=w249, "LayerID"=w249, "connection ID"=w259) -> ("error out"=w254:errorcluster, "OK?"=w251:bool, "connection ID out"=w255:refnum<k5>, "Program done"=w257:string[])  [unwired: 2 in, 1 out]
                              n57 = Index Array "Index Array"(array=w257, index=1) -> (element=w252:string)
                            }
                          }
                        }
                        frame #2 {
                          # "Crea subcarpeta d'adquisició\nper gravar els PixelReg carregats"
                          n58 = Build Path(base path=w293, name or relative path="Pixel Registers") -> (appended path=w297:path)
                          n59 = And(x=w300, y=w299) -> (x .and. y?=w285:bool)
                          n60 = call <vilib>:"Check if File or Folder Exists.vi"("path"=w297) -> ("error out"=w294:errorcluster, "file or folder exists?"=w296:bool, "dup path"=w295:path)  [unwired: 8 in]
                          n61 = case shown="False" w296 {
                            tunnel: w295 -> [w309 w310]
                            tunnel: w294 -> [w308 _]
                            tunnel: [w307 w310] -> w292
                            frame False {
                              n62 = Create Folder(path (use dialog)=w309, error in=w308) -> (created path=w307:path)  [unwired: 1 in, 2 out]
                            }
                            frame True {
                            }
                          }
                          n63 = property on="Operation text" class="Str"(reference=w305, error in=w304, "Value"="Clearing noise...\nProgramming Pixel Regs...") -> ()  [unwired: 2 out]
                        }
                        frame #3 {
                          w315 = "\r"
                          # "Si un chip no està equalitzat,\nse li programa un PixelReg defecte"
                          # "default values for acquire"
                          # "PixelReg es crea segons I Leak\n21nov2016: PxReset ON"
                          n64 = local read "Layer ID list 2 (ordered)"() -> (w328:u32[])
                          n65 = local read "Layer ID list 1 (ordered)"() -> (w335:u32[])
                          n66 = for {
                            N: 100 -> [_]
                            tunnel: w337 -> [w381]
                            tunnel: [w378] -> w319 mode=concatenating
                            workers-P: _ -> [_]
                            w385 = u8 4  # bits 34, 35
                            # "100 x PixelReg"
                            n67 = Multiply(x=w381, y=w385) -> (x*y=w383:u8)
                            n68 = To Unsigned Long Integer(number=w383) -> (unsigned 32bit integer=w382:u32)
                            n69 = Add(x=u32 384, y=w382) -> (x+y=w379:u32)
                            n70 = Build Array(u32 671965163 ("Numeric"), w379) -> (w378:u32[])
                          }
                          n71 = call "Select PA gain.vi"() -> ("PA gain selected"=w311:u8)  [unwired: 5 in]
                          n72 = local read "Chip ID list 2"() -> (w327:u32[])
                          n73 = local read "Chip ID list 1"() -> (w334:u32[])
                          n74 = local read "All ID list 2"() -> (w329:u32[])
                          n75 = local read "All ID list 1"() -> (w336:u32[])
                          n76 = case shown="True" w330 {
                            tunnel: [w363 w377] -> w325
                            tunnel: w340 -> [_ w376]
                            tunnel: w339 -> [w363 w375]
                            tunnel: [w362 w372] -> w338
                            tunnel: w319 -> [_ w371]
                            tunnel: w318 -> [_ w370]
                            tunnel: w317 -> [_ w369]
                            tunnel: [_ w368] -> w316
                            tunnel: w336 -> [_ w365]
                            tunnel: w335 -> [_ w366]
                            tunnel: w334 -> [_ w367]
                            tunnel: w331 -> [w362 _]
                            tunnel: w311 -> [_ w364]
                            frame False {
                              # "Hardware 1 not enabled"
                            }
                            frame True {
                              # "Hardware 1 enabled"
                              n77 = call "PixelReg ProgramFromFile 2nPas.vi"("connection ID"=w376, "ACQ PxReg folder"=w369, "EQ folder path"=w370, "PixelReg (hex)"=w371, "All ID list"=w365, "Layer ID list"=w366, "Chip ID list"=w367, "error in (no error)"=w375, "PA gain"=w364) -> ("connection ID out"=w374:refnum<k5>, "done message"=w368:string, "All checks OK"=w372:bool, "error out (no error)"=w373:errorcluster)  [unwired: 2 in, 1 out]
                              n78 = call "CloseEthConnection.vi"("error in (no error)"=w373, "connection ID"=w374) -> ("error out"=w377:errorcluster)  [unwired: 9 in]
                            }
                          }
                          n79 = case shown="True" w331 {
                            tunnel: [w347 w361] -> w324
                            tunnel: w333 -> [_ w360]
                            tunnel: w332 -> [w347 w359]
                            tunnel: [w346 w356] -> w322
                            tunnel: w319 -> [_ w355]
                            tunnel: w318 -> [_ w354]
                            tunnel: w317 -> [_ w353]
                            tunnel: [_ w352] -> w312
                            tunnel: w329 -> [_ w349]
                            tunnel: w328 -> [_ w350]
                            tunnel: w327 -> [_ w351]
                            tunnel: w330 -> [w346 _]
                            tunnel: w311 -> [_ w348]
                            frame False {
                              # "Hardware 2 not enabled"
                            }
                            frame True {
                              # "Hardware 2 enabled"
                              n80 = call "PixelReg ProgramFromFile 2nPas.vi"("connection ID"=w360, "ACQ PxReg folder"=w353, "EQ folder path"=w354, "PixelReg (hex)"=w355, "All ID list"=w349, "Layer ID list"=w350, "Chip ID list"=w351, "error in (no error)"=w359, "PA gain"=w348) -> ("connection ID out"=w358:refnum<k5>, "done message"=w352:string, "All checks OK"=w356:bool, "error out (no error)"=w357:errorcluster)  [unwired: 2 in, 1 out]
                              n81 = call "CloseEthConnection.vi"("error in (no error)"=w357, "connection ID"=w358) -> ("error out"=w361:errorcluster)  [unwired: 9 in]
                            }
                          }
                          n82 = Merge Errors(w325, w324) -> (w326:errorcluster)
                          n83 = call <vilib>:"Simple Error Handler.vi"("error in (no error)"=w326) -> ()  [unwired: 4 in, 5 out]
                          n84 = Unbundle By Name(w326) -> ("status"=w341:bool)
                          n85 = Concatenate Strings "Concatenate Strings"(w321, w320, w316, w315, w315, w314, w313, w312) -> (w344:string)
                          n86 = Compound Arithmetic op=AND(invert w341, w338, w323, w322) -> (w343:bool)
                          n87 = property on="Error tick" class="Bool (strict)"(reference=w342, "Value"=w341) -> ()  [unwired: 1 in, 2 out]
                          n88 = case shown="True" w343 {
                            tunnel: w344 -> [_ w387]
                            frame False {
                              # "error"
                            }
                            frame True {
                              # "OK x3"
                              n89 = call "MessageTimeOk.vi"("time (ms)"=5200, "missage"=w387) -> ()  [unwired: 4 in]
                            }
                          }
                        }
                      }
                    }
                  }
                }
                frame #1 {
                  w395 = u32 0 ("Value")
                  # "Inicialitza: 'etapa2 Waiting time' + 'Waiting time X'"
                  # "Mostra quina EQualització carrega"
                  # "Llegeix HV final value from EQ loaded"
                  # "Inicialitza variables 'actual time'"
                  # "1) Inicialitzacions a la Adquisició. Ask for comments"
                  n90 = flat-sequence {
                    tunnel: w410 -> [w423]
                    tunnel: [w422] -> w406
                    tunnel: [w421] -> w404
                    tunnel: w403 -> [w421]
                    tunnel: [w427] -> w408
                    tunnel: [w426] -> w407
                    tunnel: w406 -> [w426]
                    tunnel: w404 -> [w425]
                    tunnel: [w430] -> w405
                    tunnel: w408 -> [w430]
                    tunnel: w407 -> [w429]
                    frame #0 {
                      n91 = property on="Operation text" class="Str"(reference=w423, "Value"="Clearing noise...\nWrite comments for file.") -> (reference out=w422:refnum<vi>)  [unwired: 1 in, 1 out]
                    }
                    frame #1 {
                      # "ask for comments"
                      n92 = call "Acq_askComents.vi"("Folder path"=w425) -> ("Complete file path"=w427:path)  [unwired: 4 in]
                    }
                    frame #2 {
                      n93 = property on="Operation text" class="Str"(reference=w429, "Value"="Clearing noise...") -> ()  [unwired: 1 in, 2 out]
                    }
                  }
                  n94 = property on="etapa2 Actual time" class="DigNum (strict)"(reference=w420, "Value"=w395) -> ()  [unwired: 1 in, 2 out]
                  n95 = property on="etapa5 Actual time" class="DigNum (strict)"(reference=w418, "Value"=w395) -> ()  [unwired: 1 in, 2 out]
                  n96 = property on="Events fets" class="DigNum (strict)"(reference=w398, "Value"=w395) -> ()  [unwired: 1 in, 2 out]
                  n97 = property on="Events fets A" class="DigNum (strict)"(reference=w397, "Value"=w395) -> ()  [unwired: 1 in, 2 out]
                  n98 = property on="Events fets B" class="DigNum (strict)"(reference=w396, "Value"=w395) -> ()  [unwired: 1 in, 2 out]
                  n99 = property on="etapa3 Actual time" class="DigNum (strict)"(reference=w419, "Value"=w395) -> ()  [unwired: 1 in, 2 out]
                  n100 = property on="HV parameters" class="Clust (strict)"(reference=w417) -> (reference out=w414:refnum<vi>, "Value"=w416:T6)  [unwired: 1 in, 1 out]
                  n101 = property on="Stop ACQ button" class="Bool (strict)"(reference=w402, "Value"=FALSE, "DisabledEnum"=T5."Enabled" ("Disabled"), "Visible"=TRUE) -> ()  [unwired: 1 in, 2 out]
                  n102 = in-place {
                    in-place-border: w409 -> [w431]
                    n103 = in-place-cluster #1(w416) -> ()  [unwired: 1 out]
                    n104 = in-place-cluster #1("Final value"=w431) -> (w415:T6)
                  }
                  n105 = String To Path(string=w411) -> (path=w412:path)
                  n106 = property class="Path"(reference="EQ folder path Refnum", "Value"=w412) -> ()  [unwired: 1 in, 2 out]
                  n107 = property on="HV parameters" class="Clust (strict)"(reference=w414, "Value"=w415) -> ()  [unwired: 1 in, 2 out]
                  n108 = property on="etapa2 Waiting time" class="DigNum (strict)"(reference=w394) -> (reference out=w388:refnum<vi>, error out=w392:errorcluster, "Value"=w391:u32)  [unwired: 1 in]
                  n109 = Unbundle By Name(w393) -> ("Waiting time X"=w390:u32)
                  n110 = Add(x=w391, y=w390) -> (x+y=w389:u32)
                  n111 = property on="etapa2 Waiting time" class="DigNum (strict)"(reference=w388, error in=w392, "Value"=w389) -> ()  [unwired: 2 out]
                }
                frame #2 {
                  w436 = u32 0  # Comptador events per file
                  w440 = u32 0  # Total ACQ time
                  w443 = u32 1  # first file sufix num.
                  # "Desactiva busy per permetre\nmesura de temperatura\ndurant ACQ data viewer."
                  # "2) ADQUISICIÓ"
                  n112 = while {
                    tunnel: w463 -> [w497]
                    tunnel: w462 -> [w496]
                    tunnel: w461 -> [w495]
                    tunnel: w460 -> [w494]
                    tunnel: w459 -> [w493]
                    tunnel: w458 -> [w492]
                    tunnel: w457 -> [w491]
                    tunnel: w456 -> [w490]
                    tunnel: w455 -> [w489]
                    tunnel: w454 -> [w488]
                    tunnel: w453 -> [w487]
                    tunnel: w452 -> [w486]
                    tunnel: w451 -> [w485]
                    tunnel: w442 -> [w484]
                    tunnel: w450 -> [w483]
                    tunnel: w449 -> [w482]
                    tunnel: [w481] -> w434 mode=indexing
                    tunnel: w448 -> [w479]
                    tunnel: w447 -> [w478]
                    tunnel: w446 -> [w477]
                    tunnel: [w476] -> w444
                    shift-right: [w466] -> _
                    shift-left: w443 -> [w468]
                    tunnel: [w469] -> w441
                    shift-right: [w474] -> w439
                    shift-left: w440 -> [w475]
                    tunnel: w438 -> [w473]
                    tunnel: w437 -> [w472]
                    shift-right: [w465] -> _
                    shift-left: w436 -> [w467]
                    tunnel: w435 -> [w471]
                    tunnel: w432 -> [w464]
                    i -> [w470]
                    stop <- w480 stop-if-true
                    # "HV it"
                    n113 = stacked-sequence {
                      tunnel: w497 -> [_ _ w559 _ _ _ _]
                      tunnel: w496 -> [_ _ w561 _ _ _ _]
                      tunnel: w495 -> [w505 _ w560 _ _ _ _]
                      tunnel: w494 -> [_ _ _ w621 _ _ _]
                      tunnel: w493 -> [w504 _ _ w620 _ _ _]
                      tunnel: w492 -> [_ _ _ _ _ w807 _]
                      tunnel: w491 -> [_ _ _ _ _ w808 _]
                      tunnel: w490 -> [w503 _ _ _ _ w806 _]
                      tunnel: w489 -> [_ w517 _ _ w767 _ _]
                      tunnel: w488 -> [_ w510 _ _ w766 _ _]
                      tunnel: w487 -> [_ w513 _ w623 w765 _ _]
                      tunnel: w486 -> [_ w508 _ _ w764 _ _]
                      tunnel: w485 -> [_ w518 w558 w619 w758 w805 w852]
                      tunnel: w484 -> [_ w515 w557 _ w761 w804 _]
                      tunnel: w483 -> [_ _ _ w625 _ _ _]
                      tunnel: w482 -> [_ _ _ w624 _ _ _]
                      tunnel: [_ _ _ w622 _ _ _] -> w481
                      tunnel: [_ _ _ _ _ _ w851] -> w480
                      tunnel: w479 -> [_ _ _ w617 _ _ _]
                      tunnel: w478 -> [_ w507 w555 w605 w759 w802 w850]
                      tunnel: w477 -> [_ _ w553 _ _ w800 _]
                      tunnel: [_ _ _ _ _ _ w850] -> w476
                      tunnel: w475 -> [_ _ _ w613 _ _ _]
                      tunnel: [_ _ _ w612 _ _ _] -> w474
                      tunnel: w473 -> [_ _ _ w616 _ _ _]
                      tunnel: w472 -> [_ _ _ w615 _ _ _]
                      tunnel: w471 -> [w500 _ _ w614 _ _ _]
                      tunnel: w470 -> [w501 _ _ w607 _ _ _]
                      tunnel: [w498 _ _ _ _ _ _] -> w469
                      tunnel: w468 -> [_ _ _ w611 _ _ _]
                      tunnel: w467 -> [_ _ _ w610 _ _ _]
                      tunnel: [_ _ _ w609 _ _ _] -> w466
                      tunnel: [_ _ _ w608 _ _ _] -> w465
                      tunnel: w464 -> [_ _ _ w603 _ _ _]
                      frame #0 {
                        w502 = u8 0 ("ACQ-e2 barra")
                        # "Inicialitzacions a la iteració"
                        n114 = Increment(x=w501) -> (x+1=w498:i32)
                        n115 = Unbundle By Name(w500) -> ("HVit Refnum"=w499:refnum<vi>)
                        n116 = property on="HV it" class="DigNum (strict)"(reference=w499, "Value"=w498) -> ()  [unwired: 1 in, 2 out]
                        n117 = property on="etapa2 barra" class="Slide (strict)"(reference=w505, "Value"=w502) -> ()  [unwired: 1 in, 2 out]
                        n118 = property on="etapa3 barra" class="Slide (strict)"(reference=w504, "Value"=w502) -> ()  [unwired: 1 in, 2 out]
                        n119 = property on="etapa5 barra" class="Slide (strict)"(reference=w503, "Value"=w502) -> ()  [unwired: 1 in, 2 out]
                      }
                      frame #1 {
                        # "Etapa 1:  rampa pujada HV"
                        n120 = flat-sequence {
                          tunnel: w518 -> [w519]
                          tunnel: w517 -> [w524]
                          tunnel: [w527] -> w516
                          tunnel: w515 -> [w526]
                          tunnel: [w525] -> w514
                          tunnel: w513 -> [w525]
                          tunnel: [w524] -> w512
                          tunnel: [w523] -> w511
                          tunnel: w510 -> [w523]
                          tunnel: [w522] -> w509
                          tunnel: w508 -> [w522]
                          tunnel: w507 -> [w520]
                          tunnel: [w519] -> w506
                          frame #0 {
                            # "Desactiva busy per permetre\nmesura de temperatura\ndurant rampa HV i temps H"
                            n121 = property on="HV level" class="Slide (strict)"(reference=w524) -> ("Value"=w530:dbl)  [unwired: 1 in, 2 out]
                            n122 = property on="Stop ACQ" class="Bool (strict)"(reference=w519) -> ("Value"=w528:bool)  [unwired: 1 in, 2 out]
                            n123 = property on="busy = F" class="Bool (strict)"(reference=w520, "Value"=FALSE) -> ()  [unwired: 1 in, 2 out]
                            n124 = Not Equal To 0?(x=w530) -> (x != 0?=w529:bool)
                            n125 = Compound Arithmetic op=OR "OR"(w529, w528, invert w526) -> (w527:bool)
                          }
                        }
                        n126 = case shown="False" w516 {
                          tunnel: w511 -> [w538 _]
                          tunnel: w512 -> [w535 _]
                          tunnel: w514 -> [w534 _]
                          tunnel: w509 -> [w532 _]
                          tunnel: w506 -> [w531 _]
                          frame False {
                            n127 = flat-sequence {
                              tunnel: [w547] -> w541
                              tunnel: w538 -> [w552]
                              tunnel: [w550] -> w537
                              tunnel: [w549] -> w536
                              tunnel: w532 -> [w546]
                              frame #0 {
                                n128 = property on="HV parameters" class="Clust (strict)"(reference=w546) -> ("Value"=w547:T6)  [unwired: 1 in, 2 out]
                                n129 = property on="HV string" class="Str"(reference=w552, "Value"="HV ramping" ("HV String"), "Text.FontColor"=u32 15365376) -> (reference out=w550:refnum<vi>, error out=w549:errorcluster)  [unwired: 1 in]
                              }
                            }
                            n130 = call "HV_drive.vi"("Stop subVI Refnum"=w531, "HV level Refnum"=w535, "HV parameters"=w541) -> ("error out"=w540:errorcluster, "HV level (last value)"=w539:dbl)  [unwired: 1 in]
                            n131 = flat-sequence {
                              tunnel: w539 -> [_]
                              tunnel: w537 -> [w544]
                              tunnel: w536 -> [w543]
                              frame #0 {
                                n132 = property on="HV string" class="Str"(reference=w544, error in=w543, "Value"="HV presence!" ("HV String"), "Text.FontColor"=u32 16711680) -> ()  [unwired: 2 out]
                              }
                            }
                            n133 = Unbundle By Name(w540) -> ("status"=w533:bool)
                            n134 = call <vilib>:"Simple Error Handler.vi"("error in (no error)"=w540) -> ()  [unwired: 4 in, 5 out]
                            n135 = property on="Error tick" class="Bool (strict)"(reference=w534, "Value"=w533) -> ()  [unwired: 1 in, 2 out]
                          }
                          frame True {
                            # "executant aturada\no hi ha HV manual\no HV not enabled"
                          }
                        }
                      }
                      frame #2 {
                        # "Etapa 2:  temps inicial a HV_H"
                        n136 = flat-sequence {
                          tunnel: w561 -> [w568]
                          tunnel: w560 -> [w567]
                          tunnel: w559 -> [w566]
                          tunnel: w558 -> [w565]
                          tunnel: w557 -> [w564]
                          tunnel: [w563] -> w556
                          tunnel: w555 -> [w563]
                          tunnel: [w562] -> w554
                          tunnel: w553 -> [w562]
                          tunnel: w556 -> [w597]
                          tunnel: w554 -> [w596]
                          frame #0 {
                            n137 = case shown="True" w564 {
                              tunnel: w568 -> [_ w574]
                              tunnel: w567 -> [_ w572]
                              tunnel: w566 -> [_ w571]
                              tunnel: w565 -> [_ w570]
                              frame False {
                              }
                              frame True {
                                n138 = property on="etapa2 Actual time" class="DigNum (strict)"(reference=w574, "Value"=u32 0 ("ACQ-e2 Actual time")) -> (reference out=w573:refnum<vi>)  [unwired: 1 in, 1 out]
                                n139 = Tick Count (ms)() -> (millisecond timer value=w575:u32)
                                n140 = while {
                                tunnel: w575 -> [w594]
                                tunnel: w573 -> [w584]
                                tunnel: w571 -> [w583]
                                tunnel: w572 -> [w581]
                                tunnel: w570 -> [w577]
                                stop <- w579 stop-if-true
                                n141 = property on="etapa2 Waiting time" class="DigNum (strict)"(reference=w583) -> ("Value"=w582:u32)  [unwired: 1 in, 2 out]
                                n142 = Tick Count (ms)() -> (millisecond timer value=w595:u32)
                                n143 = property on="Stop ACQ" class="Bool (strict)"(reference=w577) -> ("Value"=w576:bool)  [unwired: 1 in, 2 out]
                                n144 = Subtract(x=w595, y=w594) -> (x-y=w593:u32)
                                n145 = Quotient & Remainder(x=w593, y=u32 1000) -> (floor(x/y)=w585:u32)  [unwired: 1 out]
                                n146 = Greater Or Equal?(x=w585, y=w582) -> (x >= y?=w578:bool)
                                n147 = To Double Precision Float(number=w585) -> (double precision float=w586:dbl)
                                n148 = To Double Precision Float(number=w582) -> (double precision float=w587:dbl)
                                n149 = property on="etapa2 Actual time" class="DigNum (strict)"(reference=w584, "Value"=w585) -> ()  [unwired: 1 in, 2 out]
                                n150 = Divide(x=w586, y=w587) -> (x/y=w590:dbl)
                                n151 = Or(x=w578, y=w576) -> (x .or. y?=w579:bool)
                                n152 = Multiply(x=w590, y=100.0) -> (x*y=w588:dbl)
                                n153 = To Unsigned Byte Integer(number=w588) -> (unsigned 8bit integer=w580:u8)
                                n154 = property on="etapa2 barra" class="Slide (strict)"(reference=w581, "Value"=w580) -> ()  [unwired: 1 in, 2 out]
                                n155 = Wait Until Next ms Multiple(millisecond multiple=u32 100) -> ()  [unwired: 1 out]
                                }
                              }
                            }
                          }
                          frame #1 {
                            # "Reactiva busy per procedir a l'adquisició"
                            n156 = flat-sequence {
                              tunnel: w597 -> [w601]
                              tunnel: w596 -> [w599]
                              tunnel: [w599] -> w598
                              tunnel: w598 -> [w602]
                              frame #0 {
                                n157 = property on="busy = T" class="Bool (strict)"(reference=w601, "Value"=TRUE) -> ()  [unwired: 1 in, 2 out]
                              }
                              frame #1 {
                                n158 = Wait (ms)(milliseconds to wait=w602) -> ()  [unwired: 1 out]
                              }
                            }
                          }
                        }
                      }
                      frame #3 {
                        # "Etapa 3:  adquisició"
                        n159 = property on="Stop ACQ button" class="Bool (strict)"(reference=w619) -> ("Value"=w618:bool)  [unwired: 1 in, 2 out]
                        n160 = property on="busy = T" class="Bool (strict)"(reference=w605, "Value"=TRUE) -> (reference out=w604:refnum<vi>)  [unwired: 1 in, 1 out]
                        n161 = case shown="False" w618 {
                          tunnel: w625 -> [w643 _]
                          tunnel: w624 -> [w641 _]
                          tunnel: w623 -> [w648 _]
                          tunnel: w619 -> [w634 _]
                          tunnel: [w637 _] -> w622
                          tunnel: w621 -> [w644 _]
                          tunnel: w620 -> [w645 _]
                          tunnel: w617 -> [w642 _]
                          tunnel: w616 -> [w640 _]
                          tunnel: w615 -> [w639 _]
                          tunnel: w614 -> [w636 _]
                          tunnel: w613 -> [w633 w757]
                          tunnel: [w632 w757] -> w612
                          tunnel: w611 -> [w631 w756]
                          tunnel: w610 -> [w630 w755]
                          tunnel: [w629 w756] -> w609
                          tunnel: [w628 w755] -> w608
                          tunnel: w607 -> [w627 _]
                          tunnel: w604 -> [_ _]
                          tunnel: w603 -> [w626 _]
                          frame False {
                            # "si no hi ha Stop ordenat, adquireix"
                            n162 = Unbundle By Name(w636) -> ("ClearNoise ACQits"=w635:i32)
                            n163 = in-place "Conversion of DTP: ms to comptes" {
                              n164 = in-place-cluster #2("ACQ Parameters (cluster)") -> ("DTP period"=w749:u32)
                              n165 = To Double Precision Float(number=w749) -> (double precision float=w750:dbl)
                              n166 = Divide(x=w750, y=2.5e-05) -> (x/y=w753:dbl)
                              n167 = Decrement(x=w753) -> (x-1=w752:dbl)
                              n168 = To Unsigned Long Integer(number=w752) -> (unsigned 32bit integer=w751:u32)
                              n169 = in-place-cluster #2("DTP period"=w751) -> (w653:T3)
                            }
                            n170 = property class="DigNum (strict)"(reference="Events to acquire Refnum") -> ("Value"=w649:u32)  [unwired: 1 in, 2 out]
                            n171 = Cluster To Array(cluster=w653) -> (array=w646:u32[])
                            n172 = Bundle(TRUE, "Value"=w649) -> (w647:cluster{bool, "Value":u32})  [unwired: 1 in]
                            n173 = for {
                              N: w635 -> [_]
                              tunnel: w648 -> [w677]
                              tunnel: w634 -> [w676]
                              tunnel: w647 -> [w675]
                              tunnel: w646 -> [w674]
                              tunnel: w645 -> [w673]
                              tunnel: w644 -> [w672]
                              tunnel: w643 -> [w671]
                              tunnel: w642 -> [w670]
                              tunnel: [w666] -> w638 mode=indexing
                              tunnel: w641 -> [w669]
                              tunnel: w640 -> [w668]
                              tunnel: w639 -> [w667]
                              tunnel: w636 -> [w665]
                              shift-right: [w663] -> w632
                              shift-left: w633 -> [w664]
                              shift-right: [w660] -> w629
                              shift-left: w631 -> [w662]
                              shift-right: [w659] -> w628
                              shift-left: w630 -> [w661]
                              tunnel: w627 -> [w658]
                              tunnel: w626 -> [w654]
                              i -> [w655]
                              stop <- w657 stop-if-true
                              # "ACQ it"
                              n174 = Increment(x=w655) -> (x+1=w656:i32)
                              n175 = stacked-sequence {
                                tunnel: w677 -> [_ w698 _ _]
                                tunnel: w676 -> [_ w695 _ w731]
                                tunnel: w675 -> [_ w694 _ _]
                                tunnel: w674 -> [_ w693 _ _]
                                tunnel: w673 -> [_ w692 _ _]
                                tunnel: w672 -> [_ w691 w710 _]
                                tunnel: w671 -> [_ w690 _ _]
                                tunnel: w670 -> [_ w689 _ _]
                                tunnel: w669 -> [_ w684 _ w722]
                                tunnel: w668 -> [_ w683 _ _]
                                tunnel: w667 -> [_ w682 _ _]
                                tunnel: [_ w681 _ _] -> w666
                                tunnel: w665 -> [w680 _ _ w723]
                                tunnel: w656 -> [w678 _ _ w741]
                                tunnel: w664 -> [_ _ w709 _]
                                tunnel: [_ _ w708 _] -> w663
                                tunnel: w662 -> [_ _ _ w740]
                                tunnel: w661 -> [_ _ _ w739]
                                tunnel: [_ _ _ w713] -> w660
                                tunnel: [_ _ _ w712] -> w659
                                tunnel: w658 -> [_ _ _ w744]
                                tunnel: [_ _ _ w725] -> w657
                                tunnel: w654 -> [_ _ _ w716]
                                frame #0 {
                                # "inicialitzacions"
                                n176 = Unbundle By Name(w680) -> ("ACQit Refnum"=w679:refnum<vi>)
                                n177 = property on="ACQ it" class="DigNum (strict)"(reference=w679, "Value"=w678) -> ()  [unwired: 1 in, 2 out]
                                }
                                frame #1 {
                                # "Adquisició"
                                n178 = local read "Addresses Cluster"() -> (w685:T2)
                                n179 = local read "LayerChipIDs"() -> (w700:u16[])
                                n180 = call "subop_x2_Acquisition.vi"("ACQ stop by events"=w694, "LayerChipIDs"=w700, "ACQ parameters"=w693, "events fets A Refnum"=w683, "events fets B Refnum"=w682, "Base file path"=w684, "Addresses Cluster"=w685, "Stop ACQ button Refnum"=w695, "ACQ barra Refnum"=w692, "Actual time Refnum"=w691, "Acquisition time Refnum"=w690, "Total events Refnum"=w689) -> ("ACQ WatchDog timeout"=w681:bool, "ACQ Answer 1i2"=w686:string, "error out comm"=w688:errorcluster, "error out file"=w687:errorcluster)  [unwired: 11 in, 1 out]
                                n181 = Merge Errors(w688, w687) -> (w699:errorcluster)
                                n182 = Or(x=w687, y=w681) -> (x .or. y?=w696:bool)
                                n183 = call <vilib>:"Simple Error Handler.vi"("error in (no error)"=w699) -> ()  [unwired: 4 in, 5 out]
                                n184 = Unbundle By Name(w699) -> ("status"=w697:bool)
                                n185 = case shown="False" w696 {
                                tunnel: w686 -> [w703 _]
                                frame False {
                                # "No hi ha errors file"
                                n186 = Concatenate Strings(w703, "\r", "The files have been saved.") -> (w706:string)
                                n187 = call "MessageTimeOk.vi"("time (ms)"=3500, "missage"=w706) -> ()  [unwired: 4 in]
                                }
                                frame True {
                                # "Algun error"
                                }
                                }
                                n188 = case shown="True" w681 {
                                frame False {
                                }
                                frame True {
                                n189 = call "MessageTimeOk.vi"("time (ms)"=10000, "missage"="Acquisition WatchDog timeout." ("message")) -> ()  [unwired: 4 in]
                                }
                                }
                                n190 = property on="Error tick" class="Bool (strict)"(reference=w698, "Value"=w697) -> ()  [unwired: 1 in, 2 out]
                                }
                                frame #2 {
                                n191 = property on="etapa3 Actual time (ACQ time)" class="DigNum (strict)"(reference=w710) -> ("Value"=w711:u32)  [unwired: 1 in, 2 out]
                                n192 = Add(x=w711, y=w709) -> (x+y=w708:u32)
                                }
                                frame #3 {
                                # "analisis +"
                                n193 = Unbundle By Name(w723) -> ("Threshold Z"=w724:u32, "ClearNoise ACQits"=w743:i32)
                                n194 = local read "Chip ID list 1"() -> (w737:u32[])
                                n195 = local read "Chip ID list 2"() -> (w736:u32[])
                                n196 = local read "Addresses Cluster"() -> (w738:T2)
                                n197 = To Unsigned Word Integer(number=w736) -> (unsigned 16bit integer=w732:u16[])
                                n198 = To Unsigned Word Integer(number=w737) -> (unsigned 16bit integer=w733:u16[])
                                n199 = Multiply(x=w743, y=w744) -> (x*y=w742:i32)
                                n200 = Add(x=w742, y=w741) -> (x+y=w745:i32)
                                n201 = call "ACQ PostProces1.vi"("ACQ full DATA file path"=w722, "Addresses Cluster"=w738, "Chip ID list 2"=w732, "Chip ID list 1"=w733, "events per file in"=w739, "file sufix num. in"=w740) -> ("summary temp B"=w734:u32[][], "summary temp A"=w735:u32[][], "events per file out"=w712:u32, "file sufix num. out"=w713:u32)  [unwired: 2 in]
                                n202 = local read "Layer ID list 2 (ordered)"() -> (w721:u32[])
                                n203 = local read "Layer ID list 1 (ordered)"() -> (w719:u32[])
                                n204 = local read "Addresses Cluster"() -> (w717:T2)
                                n205 = call "ClearNoise analisis.vi"("summary temp A"=w735, "summary temp B"=w734, "Chip ID list 1"=w733, "Chip ID list 2"=w732, "Threshold Z"=w724) -> ("Killing list A"=w715:T7, "Killing list B"=w714:T7)
                                n206 = local read "All ID list 2"() -> (w720:u32[])
                                n207 = local read "All ID list 1"() -> (w718:u32[])
                                n208 = property on="Stop ACQ button" class="Bool (strict)"(reference=w731) -> (reference out=w726:refnum<vi>, "Value"=w730:bool)  [unwired: 1 in, 1 out]
                                n209 = call "ClearNoise Log.vi"("ACQ full DATA file path"=w722, "Log it"=w745, "ClearNoise vars"=w723, "Killing list B"=w714, "Killing list A"=w715) -> ()  [unwired: 7 in]
                                n210 = Empty Array? "Empty Arrays?"(array=w715) -> (empty?=w729:bool)
                                n211 = Empty Array?(array=w714) -> (empty?=w728:bool)
                                n212 = And(x=w729, y=w728) -> (x .and. y?=w727:bool)
                                n213 = call "Kill pixels +Program.vi"("Layer ID list 2 (ordered)"=w721, "All ID list 2"=w720, "Layer ID list 1 (ordered)"=w719, "All ID list 1"=w718, "Addresses Cluster"=w717, "ACQ full DATA file path"=w722, "EQ folder path"=w716, "Killing list A"=w715, "Killing list B"=w714) -> ()  [unwired: 11 in]
                                n214 = Or(x=w727, y=w730) -> (x .or. y?=w725:bool)
                                n215 = case shown="True" w725 {
                                selector: w725 -> [_ w746]
                                tunnel: w726 -> [_ w747]
                                frame False {
                                }
                                frame True {
                                n216 = property on="Stop ACQ button" class="Bool (strict)"(reference=w747, "Value"=w746, "DisabledEnum"=T5."Disabled" ("Disabled")) -> ()  [unwired: 1 in, 2 out]
                                }
                                }
                                }
                              }
                            }
                            n217 = And Array Elements(Boolean array=w638) -> (logical AND=w637:bool)
                          }
                          frame True {
                            # "Stop ordenat"
                          }
                        }
                      }
                      frame #4 {
                        # "Tant si hi ha Stop adquisició ordenat com si no, executa rampa baixada HV"
                        # "Etapa 4:  rampa bajada HV"
                        n218 = flat-sequence {
                          tunnel: w761 -> [w771]
                          tunnel: [w771] -> w760
                          tunnel: w759 -> [w769]
                          frame #0 {
                            # "Desactiva busy per permetre\nmesura de temperatura\ndurant rampa HV i temps L"
                            n219 = property on="busy = F" class="Bool (strict)"(reference=w769, "Value"=FALSE) -> ()  [unwired: 1 in, 2 out]
                          }
                        }
                        n220 = property on="HV level" class="Slide (strict)"(reference=w767) -> ("Value"=w768:dbl)  [unwired: 1 in, 2 out]
                        n221 = Not Equal To 0?(x=w768) -> (x != 0?=w763:bool)
                        n222 = And(x=w763, y=w760) -> (x .and. y?=w762:bool)
                        n223 = case shown="True" w762 {
                          tunnel: w767 -> [_ w776]
                          tunnel: w766 -> [_ w775]
                          tunnel: w765 -> [_ w774]
                          tunnel: w764 -> [_ w773]
                          tunnel: w758 -> [_ w772]
                          frame False {
                            # "HV = 0,   no cal baixada"
                          }
                          frame True {
                            n224 = flat-sequence {
                              tunnel: [w793] -> w777
                              tunnel: w775 -> [w799]
                              tunnel: [w797] -> w780
                              tunnel: [w796] -> w781
                              tunnel: w773 -> [w794]
                              frame #0 {
                                n225 = property on="HV parameters" class="Clust (strict)"(reference=w794) -> ("Value"=w793:T6)  [unwired: 1 in, 2 out]
                                n226 = property on="HV string" class="Str"(reference=w799, "Value"="HV ramping" ("HV String"), "Text.FontColor"=u32 15365376) -> (reference out=w797:refnum<vi>, error out=w796:errorcluster)  [unwired: 1 in]
                              }
                            }
                            n227 = call "HV_drive.vi"("Stop subVI Refnum"=w772, "HV level Refnum"=w776, "HV parameters"=w777) -> ("error out"=w778:errorcluster, "HV level (last value)"=w779:dbl)  [unwired: 1 in]
                            n228 = flat-sequence {
                              tunnel: w779 -> [w785]
                              tunnel: w780 -> [w792]
                              tunnel: w781 -> [w791]
                              frame #0 {
                                n229 = Equal To 0?(x=w785) -> (x = 0?=w790:bool)
                                n230 = Select(t="HV off", s=w790, f="HV presence!") -> (s? t:f=w784:string)
                                n231 = Select(t=u32 42533, s=w790, f=u32 16711680) -> (s? t:f=w783:u32)
                                n232 = property on="HV string" class="Str"(reference=w792, error in=w791, "Value"=w784, "Text.FontColor"=w783) -> ()  [unwired: 2 out]
                              }
                            }
                            n233 = Unbundle By Name(w778) -> ("status"=w782:bool)
                            n234 = call <vilib>:"Simple Error Handler.vi"("error in (no error)"=w778) -> ()  [unwired: 4 in, 5 out]
                            n235 = property on="Error tick" class="Bool (strict)"(reference=w774, "Value"=w782) -> ()  [unwired: 1 in, 2 out]
                          }
                        }
                      }
                      frame #5 {
                        # "Etapa 5:  temps final a HV_L"
                        n236 = flat-sequence {
                          tunnel: w808 -> [w815]
                          tunnel: w807 -> [w814]
                          tunnel: w806 -> [w813]
                          tunnel: w805 -> [w812]
                          tunnel: w804 -> [w811]
                          tunnel: [w810] -> w803
                          tunnel: w802 -> [w810]
                          tunnel: [w809] -> w801
                          tunnel: w800 -> [w809]
                          tunnel: w803 -> [w844]
                          tunnel: w801 -> [w843]
                          frame #0 {
                            n237 = case shown="True" w811 {
                              tunnel: w815 -> [_ w822]
                              tunnel: w814 -> [_ w819]
                              tunnel: w813 -> [_ w818]
                              tunnel: w812 -> [_ w817]
                              frame False {
                              }
                              frame True {
                                n238 = property on="etapa5 Actual time" class="DigNum (strict)"(reference=w822, "Value"=u32 0 ("ACQ-e2 Actual time")) -> (reference out=w820:refnum<vi>)  [unwired: 1 in, 1 out]
                                n239 = Tick Count (ms)() -> (millisecond timer value=w821:u32)
                                n240 = while {
                                tunnel: w821 -> [w841]
                                tunnel: w820 -> [w831]
                                tunnel: w819 -> [w830]
                                tunnel: w818 -> [w828]
                                tunnel: w817 -> [w824]
                                stop <- w826 stop-if-true
                                # "et5: temps final a HV_L"
                                n241 = property on="etapa5 Waiting time" class="DigNum (strict)"(reference=w830) -> ("Value"=w829:u32)  [unwired: 1 in, 2 out]
                                n242 = Tick Count (ms)() -> (millisecond timer value=w842:u32)
                                n243 = property on="Stop ACQ" class="Bool (strict)"(reference=w824) -> ("Value"=w823:bool)  [unwired: 1 in, 2 out]
                                n244 = Subtract(x=w842, y=w841) -> (x-y=w840:u32)
                                n245 = Quotient & Remainder(x=w840, y=u32 1000) -> (floor(x/y)=w832:u32)  [unwired: 1 out]
                                n246 = Greater Or Equal?(x=w832, y=w829) -> (x >= y?=w825:bool)
                                n247 = To Double Precision Float(number=w832) -> (double precision float=w833:dbl)
                                n248 = To Double Precision Float(number=w829) -> (double precision float=w834:dbl)
                                n249 = property on="etapa5 Actual time" class="DigNum (strict)"(reference=w831, "Value"=w832) -> ()  [unwired: 1 in, 2 out]
                                n250 = Or(x=w825, y=w823) -> (x .or. y?=w826:bool)
                                n251 = Divide(x=w833, y=w834) -> (x/y=w837:dbl)
                                n252 = Multiply(x=w837, y=100.0) -> (x*y=w835:dbl)
                                n253 = To Unsigned Byte Integer(number=w835) -> (unsigned 8bit integer=w827:u8)
                                n254 = property on="etapa5 barra" class="Slide (strict)"(reference=w828, "Value"=w827) -> ()  [unwired: 1 in, 2 out]
                                n255 = Wait Until Next ms Multiple(millisecond multiple=u32 100) -> ()  [unwired: 1 out]
                                }
                              }
                            }
                          }
                          frame #1 {
                            # "Reactiva busy per seguir amb la seqüència"
                            n256 = flat-sequence {
                              tunnel: w844 -> [w848]
                              tunnel: w843 -> [w846]
                              tunnel: [w846] -> w845
                              tunnel: w845 -> [w849]
                              frame #0 {
                                n257 = property on="busy = T" class="Bool (strict)"(reference=w848, "Value"=TRUE) -> ()  [unwired: 1 in, 2 out]
                              }
                              frame #1 {
                                n258 = Wait (ms)(milliseconds to wait=w849) -> ()  [unwired: 1 out]
                              }
                            }
                          }
                        }
                      }
                      frame #6 {
                        # "aturar adquisició?"
                        n259 = property on="Stop ACQ" class="Bool (strict)"(reference=w852) -> ("Value"=w851:bool)  [unwired: 1 in, 2 out]
                      }
                    }
                  }
                  n260 = And Array Elements(Boolean array=w434) -> (logical AND=w433:bool)
                  n261 = property on="busy = F" class="Bool (strict)"(reference=w444, "Value"=FALSE) -> ()  [unwired: 1 in, 2 out]
                }
                frame #3 {
                  w856 = FALSE ("Value")
                  # "3) Finalització a l'adquisició"
                  n262 = property on="Stop ACQ button" class="Bool (strict)"(reference=w857, "Visible"=w856, "Value"=w856, "DisabledEnum"=T5."Enabled" ("Disabled")) -> ()  [unwired: 1 in, 2 out]
                  n263 = property on="etapa2 Waiting time" class="DigNum (strict)"(reference=w854, "Value"=w853) -> ()  [unwired: 1 in, 2 out]
                }
                frame #4 {
                  # "4) Open DATA viewer"
                  n264 = local read "ACQ Parameters (cluster)"() -> (w873:T3)
                  n265 = property on="ACQ events fets" class="DigNum (strict)"(reference=w864) -> ("Value"=w875:u32)  [unwired: 1 in, 2 out]
                  n266 = property on="etapa2 Waiting time (s)" class="DigNum (strict)"(reference=w860) -> ("Value"=w872:u32)  [unwired: 1 in, 2 out]
                  n267 = property on="etapa5 Waiting time (s)" class="DigNum (strict)"(reference=w861) -> ("Value"=w871:u32)  [unwired: 1 in, 2 out]
                  n268 = property on="Acquisition time (s)" class="DigNum (strict)"(reference=w862) -> ("Value"=w870:u32)  [unwired: 1 in, 2 out]
                  n269 = local read "GbReg params"() -> (w876:u8[])
                  n270 = property on="HV parameters" class="Clust (strict)"(reference=w863) -> ("Value"=w874:T6)  [unwired: 1 in, 2 out]
                  n271 = Index Array "Index Array"(array=w876) -> (element #1=w869:u8, element #2=w868:u8)  [unwired: 2 in]
                  n272 = call "Grava_conditionsACQ.vi"("ACQ Parameters (cluster)"=w873, "HV parameters"=w874, "ACQ events fets"=w875, "EQ folder path"=w865, "ACQ folder path"=w866, "EQ loaded?"=w867, "etapa2 Waiting time (s)"=w872, "ACQ anVref low"=w869, "Acquisition time (s)"=w870, "ACQ GbTHLD"=w868, "etapa5 Waiting time (s)"=w871, "HV loops"=w859, "Total ACQ time (s)"=w858) -> ()  [unwired: 7 in]
                  n273 = disable-structure shown="Disabled" {
                    disable-tunnel: w880 -> [w885 _]
                    disable-tunnel: w879 -> [w884 _]
                    disable-tunnel: w878 -> [w883 _]
                    disable-tunnel: w864 -> [w882 _]
                    disable-tunnel: w877 -> [w881 _]
                    frame Disabled {
                      # "Eliminar si funciona"
                      n274 = case shown="False" w885 {
                        tunnel: w884 -> [w893 _]
                        tunnel: w883 -> [w892 _]
                        tunnel: w882 -> [w891 _]
                        tunnel: w881 -> [w887 _]
                        frame False {
                          # "No hi ha timeout: obre DATA viewer"
                          n275 = flat-sequence {
                            tunnel: w891 -> [w899]
                            tunnel: w892 -> [w900]
                            tunnel: w893 -> [w901]
                            tunnel: [w901] -> w890
                            tunnel: [w900] -> w889
                            tunnel: [w899] -> w888
                            tunnel: w887 -> [w898]
                            tunnel: [w894] -> w886
                            tunnel: w890 -> [w909]
                            tunnel: w889 -> [w913]
                            tunnel: w888 -> [w912]
                            tunnel: w886 -> [w910]
                            frame #0 {
                              n276 = local read "Chip ID list 1"() -> (w896:u32[])
                              n277 = local read "Chip ID list 2"() -> (w895:u32[])
                              n278 = property on="Operation text" class="Str"(reference=w898, "Value"="Clearing noise...\nData viewer open") -> ()  [unwired: 1 in, 2 out]
                              n279 = Build Array (concatenate) "Concatenate"(w896, w895) -> (w894:u32[])
                            }
                            frame #1 {
                              n280 = Strip Path(path=w909) -> (stripped path=w908:path)  [unwired: 1 out]
                              n281 = List Folder(path=w908, pattern="*.dat") -> (filenames=w906:string[])  [unwired: 2 in, 3 out]
                              n282 = Array Size(array=w906) -> (size(s)=w905:i32)
                              n283 = for {
                                N: w905 -> [_]
                                tunnel: w910 -> [w921]
                                tunnel: w909 -> [w923]
                                shift-right: [w925] -> _
                                shift-left: w905 -> [w926]
                                tunnel: [w924] -> w903
                                tunnel: [w922] -> w904
                                tunnel: [w921] -> w902
                                n284 = To Unsigned Long Integer(number=w926) -> (unsigned 32bit integer=w927:u32)
                                n285 = Decrement(x=w926) -> (x-1=w925:i32)
                                n286 = call "Grava_summaryACQ.vi"("sufix number"=w927, "ChipID list"=w921, "ACQ full DATA file path"=w923) -> ("quants events per chip"=w924:u32[], "suffixed file path"=w922:path)  [unwired: 1 in]
                              }
                              n287 = property class="DigNum (strict)"(reference=w912) -> ("Value"=w911:u32)  [unwired: 1 in, 2 out]
                              n288 = case shown="1" w905 {
                                tunnel: w913 -> [_ w920]
                                tunnel: w911 -> [_ w919]
                                tunnel: w904 -> [_ w918]
                                tunnel: w903 -> [_ w916]
                                tunnel: w902 -> [_ w917]
                                frame Default {
                                # "Empty file path\nEmpty ChipID list"
                                # "to choose ACQ file"
                                n289 = call "ACQ_Data_viewer (Module).vi"("ACQ full DATA file path"=path "", "ChipID list"=u32[] []) -> ()  [unwired: 14 in]
                                }
                                frame 1 {
                                # "only one ACQ file"
                                n290 = call "ACQ_Data_viewer (Module).vi"("ACQ full DATA file path"=w918, "ChipID list"=w917, "quants events per chip"=w916, "ID summary"=w920, "ACQ events fets"=w919) -> ()  [unwired: 11 in]
                                }
                              }
                            }
                          }
                        }
                        frame True {
                        }
                      }
                    }
                    frame Enabled {
                      # "Obrir Data viewer condicionat"
                    }
                  }
                }
              }
            }
          }
        }
      }
    }
    frame True {
      # "connection not working"
      n291 = property on="Error tick" class="Bool (strict)"(reference=w953, "Value"=w954) -> ()  [unwired: 1 in, 2 out]
      n292 = One Button Dialog(message="The connection is NOT WORKING.\n\nCheck the wiring connection and the IP address.") -> ()  [unwired: 1 in, 1 out]
    }
  }
  "Folder path: acquisition reports" <- w1
